vi "Cell Status Data File Functions.vi"(0 "FilePathIn":path=path "C:/ER2007/Cell Status.dat", 1 "Function":T3(ring), 2 "Cell Select - RO":i32, 3 "Keys":u16(ring) items=["Title", "Version", "Last Write", "CurCell", "NumCells", "Cell ID", "Status", "Project", "Sample ID", "Rock Type", "Fluid Pair", "Rw", "Rw Temp", "Length", "Diameter", "Porosity", "Permeability", "2P/4P", "Elect Spacing", "Frequency", "Amplitude", "DAQ Period", "DAQ Units", "Start Time", "Next Time", "Filename", "Pore Volume", "Pore Transducer", "Last Resistor", "ER 1-2", "ER 1-3", "ER 1-4", "ER 2-3", "FF 2-3", "Temp A", "Temp B", "Conf Press", "Pore Press", "Delta Press", "Pore Down"], 5 "Cell x Data In":T2 {"Rw Temp" format="%.2f"; "Rw" format="%.2f"; "DAQ Units" items=["Mins", "Hrs"]; "CurData" format="%.3f"; "Last Pore Vol" format="%.3f"; "Amplitude" format="%.3f"; "ElectSpace" format="%.2f"; "Permeability" format="%.2f"; "Porosity" format="%.2f"; "Diameter" format="%.2f"; "Length" format="%.2f"}, 7 "Cell ID List":i32[](array[numeric]), 11 "ErrorIn":errorcluster, 12 "Init w Values":bool, 13 "Version":string="1.00", 14 "Sections":u16(ring) items=["GenInfo", "Cell 1 Status", "Cell 2 Status", "Cell 3 Status", "Cell 4 Status", "Cell 5 Status"]) -> (4 "FilePathOut":path=path "C:/ER2007/Cell Status.dat", 6 "Cell x Data Out":T2 {"Rw Temp" format="%.2f"; "Rw" format="%.2f"; "DAQ Units" items=["Mins", "Hrs"]; "CurData" format="%.3f"; "Last Pore Vol" format="%.3f"; "Amplitude" format="%.3f"; "ElectSpace" format="%.2f"; "Permeability" format="%.2f"; "Porosity" format="%.2f"; "Diameter" format="%.2f"; "Length" format="%.2f"}, 8 "GenInfoOut":T1, 10 "Section Strings":string[](array[string])=["GenInfo", "Cell 1 Status", "Cell 2 Status", "Cell 3 Status", "Cell 4 Status", "Cell 5 Status"], 15 "ErrorOut":errorcluster)   [LabVIEW 2013]
uses:
  <vilib>/Utility/config.llb/Write Key (String).vi
  <vilib>/Utility/config.llb/Read Key (String).vi
  <vilib>/Utility/config.llb/NI_LVConfig.lvlib
panel:
  in  "Chop Keys at Index":i32=40
  out "Labels":string[](array[string])=["Cell ID", "Status", "Project", "Sample ID", "Rock Type", "Fluid Pair", "Rw", "Rw Temp", "Length", "Diameter", "Porosity", "Permeability", "2P/4P", "Elect Spacing", "Frequency", "Amplitude", "DAQ Period", "DAQ Units", "Start Time", "Next Time", "Filename", "Pore Volume", "Pore Transducer", "Last Resistor", " ER 1-2", "ER 1-3", "ER 1-4", "ER 2-3", "FF 2-3", "Temp A", "Temp B", "Conf Press", "Pore Press", "Delta Press", "Pore Down"]
  out "ErrorOut 2":errorcluster
  in  "SetStrings":bool
  # "Specific to ER2007 Cell Status Functions"
  # "To set the strings, the file must not exist.\nSet Function to \"New File\", \"Set Strings\"\nto ON, and run vi.  After running, make\ncurrent values default for \"Sections\",\n\"Keys\", and \"Section Strings\"."
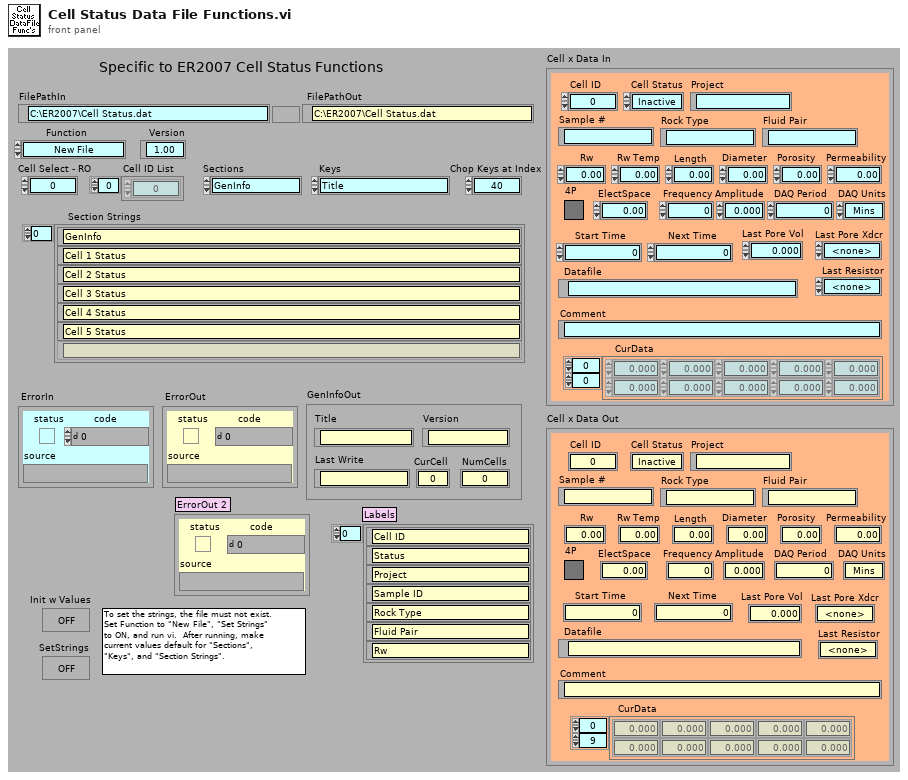
[diagram p1: front panel]
types:
  T1 = cluster{"Title":string, "Version":string, "Last Write":string, "CurCell":i32, "NumCells":i32}
  T2 = cluster{"Cell ID":i32, "Cell Status":enum16{"Inactive", "Setup", "Active", "Done"}, "Project":string, "Sample #":string, "Rock Type":string, "Fluid Pair":string, "Rw":dbl, "Rw Temp":dbl, "Length":dbl, "Diameter":dbl, "Porosity":dbl, "Permeability":dbl, "4P":bool, "ElectSpace":dbl, "Frequency":dbl, "Amplitude":dbl, "DAQ Period":u32, "DAQ Units":u16, "Start Time":dbl, "Next Time":dbl, "Datafile":path, "Last Pore Vol":dbl, "Last Pore Xdcr":enum16{"<none>", "Lo Range", "Hi Range"}, "Last Resistor":enum16{"<none>", "Resistor 1", "Resistor 2", "Resistor 3", "Resistor 4", "Resistor 5", "Resistor 6"}, "CurData":dbl[][], "Comment":string}
  T3 = enum16{"New File", "Read Cell Status", "Write Cell Status"}
  T4 = enum16{"<none>", "Resistor 1", "Resistor 2", "Resistor 3", "Resistor 4", "Resistor 5", "Resistor 6"}
  T5 = typedef "NI_LVConfig.lvlib/Config Data RefNum.ctl" = refnum<k1>
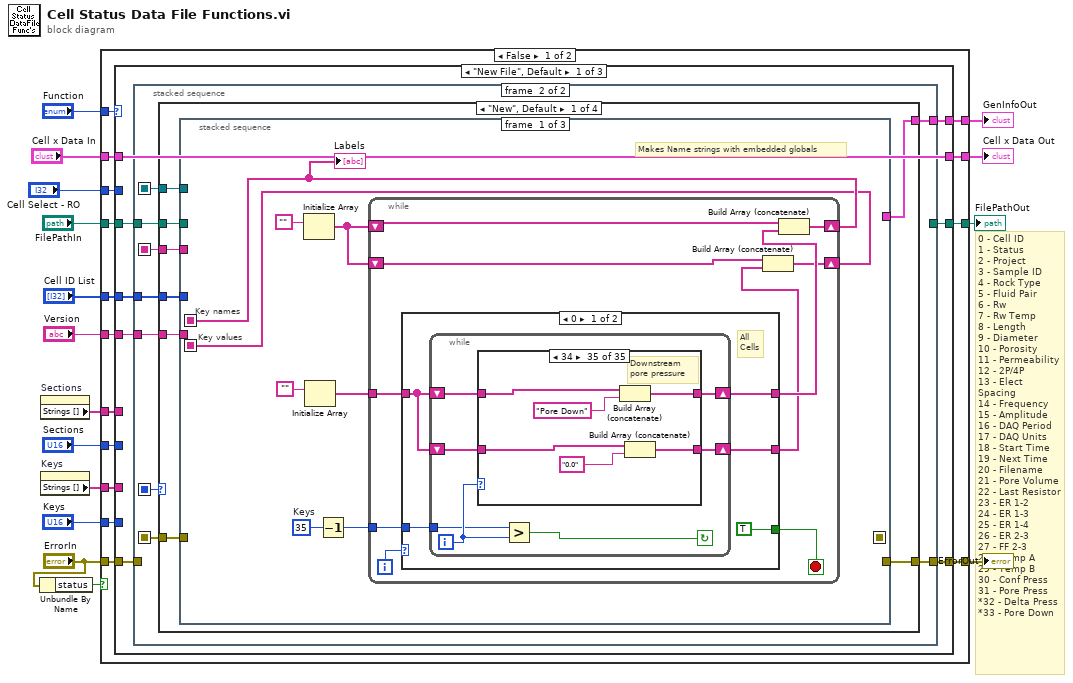
[diagram p0: block diagram]
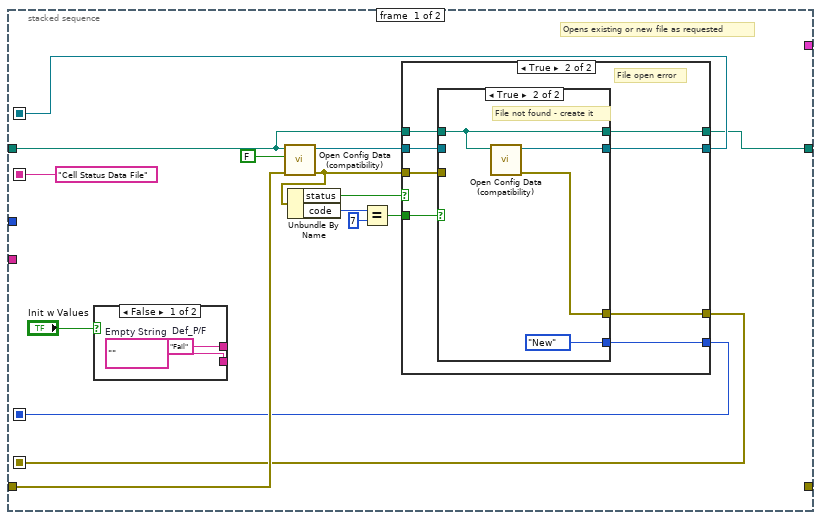
[diagram p2: hidden frame]
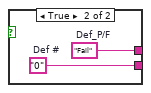
[diagram p3: hidden frame]
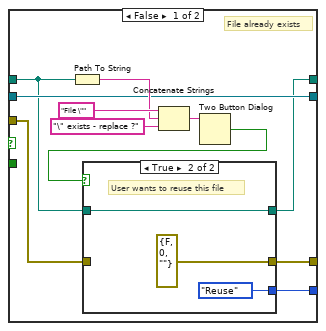
[diagram p4: hidden frame]
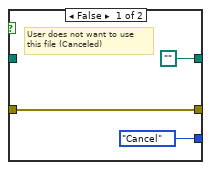
[diagram p5: hidden frame]
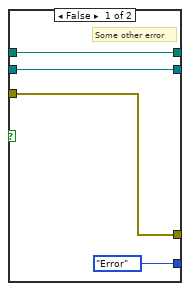
[diagram p6: hidden frame]
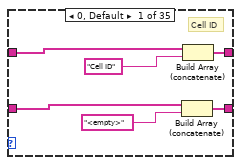
[diagram p7: hidden frame]
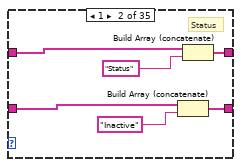
[diagram p8: hidden frame]
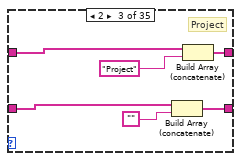
[diagram p9: hidden frame]
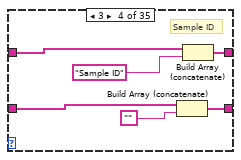
[diagram p10: hidden frame]
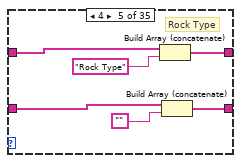
[diagram p11: hidden frame]
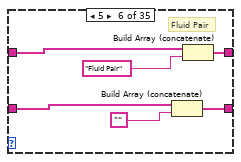
[diagram p12: hidden frame]
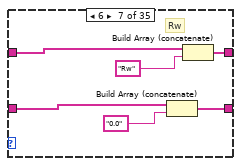
[diagram p13: hidden frame]
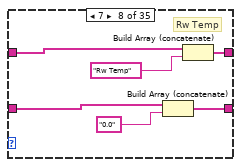
[diagram p14: hidden frame]
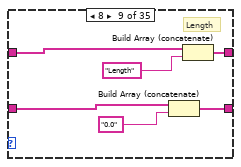
[diagram p15: hidden frame]
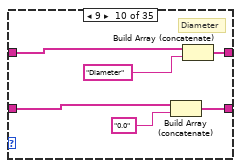
[diagram p16: hidden frame]
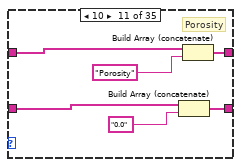
[diagram p17: hidden frame]
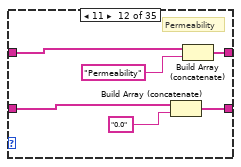
[diagram p18: hidden frame]
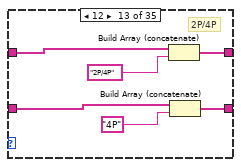
[diagram p19: hidden frame]
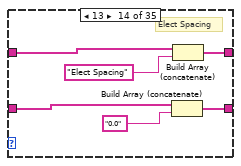
[diagram p20: hidden frame]
diagram:
  # "0 - Cell ID\n1 - Status\n2 - Project\n3 - Sample ID\n4 - Rock Type\n5 - Fluid Pair\n6 - Rw\n7 - Rw Temp\n8 - Length\n9 - Diameter\n10 - Porosity\n11 - Permeability\n12 - 2P/4P\n13 - Elect Spacing\n14 - Frequency\n15 - Amplitude\n16 - DAQ Period\n17 - DAQ Units\n18 - Start Time\n19 - Next Time\n20 - Filename\n21 - Pore Volume\n22 - Last Resistor\n23 - ER 1-2\n24 - ER 1-3\n25 - ER 1-4\n26 - ER 2-3\n27 - FF 2-3\n28 - Temp A\n29 - Temp B\n30 - Conf Press\n31 - Pore Press\n*32 - Delta Press\n*33 - Pore Down"
  n1 = Unbundle By Name("ErrorIn") -> ("status"=w16:bool)
  n2 = property on="Sections" class="Ring (strict)"() -> ("Strings []"=w11:string[])  [unwired: 2 in, 2 out]
  n3 = property on="Keys" class="Ring (strict)"() -> ("Strings []"=w9:string[])  [unwired: 2 in, 2 out]
  n4 = case shown="False" w16 {
    tunnel: "ErrorIn" -> [w29 w2061]
    tunnel: [w28 w2061] -> w14
    tunnel: "Function" -> [w31 _]
    tunnel: "FilePathIn" -> [w30 w2060]
    tunnel: "Cell ID List" -> [w27 _]
    tunnel: w11 -> [w26 _]
    tunnel: "Sections" -> [w25 _]
    tunnel: w9 -> [w24 _]
    tunnel: "Keys" -> [w23 _]
    tunnel: [w20 w2059] -> w4
    tunnel: [w22 w2060] -> w7
    tunnel: "Version" -> [w21 _]
    tunnel: "Cell x Data In" -> [w19 w2059]
    tunnel: "Cell Select - RO" -> [w18 _]
    tunnel: [w17 w2058] -> w1
    frame False {
      n5 = case shown="\"New File\", Default" w31 {
        tunnel: w30 -> [w39 w565 w1601]
        tunnel: w29 -> [w38 w577 w1612]
        tunnel: [w37 w573 w1609] -> w28
        tunnel: w27 -> [w36 _ _]
        tunnel: w26 -> [_ w567 w1604]
        tunnel: w25 -> [_ _ _]
        tunnel: w24 -> [_ w575 w1593]
        tunnel: w23 -> [_ _ _]
        tunnel: [w35 w565 w1601] -> w22
        tunnel: w21 -> [w34 _ w1592]
        tunnel: [w33 w557 w1591] -> w20
        tunnel: w19 -> [w33 w558 w1591]
        tunnel: w18 -> [_ w554 _]
        tunnel: [w32 w552 w1590] -> w17
        frame "New File", Default {
          n6 = stacked-sequence {
            seq-local: [w46 _] -> [_ w99]
            seq-local: [w44 _] -> [_ w98]
            seq-local: [w43 _] -> [_ w100]
            seq-local: ["Cell Status Data File" _] -> [_ w93]
            tunnel: w39 -> [w50 w95]
            tunnel: w38 -> [w53 _]
            tunnel: [_ w96] -> w37
            tunnel: w36 -> [_ w97]
            tunnel: [w42 _] -> w35
            tunnel: w34 -> [_ w94]
            tunnel: [_ w92] -> w32
            frame #0 {
              # "Opens existing or new file as requested"
              n7 = case shown="False" "Init w Values" {
                tunnel: [w56 w58] -> _
                tunnel: [w55 w57] -> _
                frame False {
                  w55 = ""  # Empty String
                  w56 = "Fail"  # Def_P/F
                }
                frame True {
                  w57 = "0"  # Def #
                  w58 = "Fail"  # Def_P/F
                }
              }
              n8 = call <vilib>:"Open Config Data (compatibility).vi"("error in (no error)"=w53, "create file if necessary (T)"=FALSE ("create file if necessary? (T)"), "configuration file path"=w50) -> ("error out"=w45:errorcluster, "refnum"=w51:T5)  [unwired: 6 in, 1 out]
              n9 = Unbundle By Name(w45) -> ("status"=w52:bool, "code"=w48:i32)
              n10 = Equal?(x=w48, y=7) -> (x = y?=w47:bool)
              n11 = case shown="True" w52 {
                tunnel: w51 -> [w62 w83]
                tunnel: w50 -> [w59 w78]
                tunnel: w47 -> [_ w79]
                tunnel: [w62 w82] -> w46
                tunnel: [w64 w80] -> w44
                tunnel: w45 -> [w63 w81]
                tunnel: [w61 w77] -> w43
                tunnel: [w60 w76] -> w42
                frame False {
                  # "File already exists"
                  n12 = Path To String(path=w59) -> (string=w68:string)
                  n13 = Concatenate Strings("File \"" ("message"), w68, "\" exists - replace ?" ("Substring")) -> (w66:string)
                  n14 = Two Button Dialog(message=w66) -> (T button?=w65:bool)  [unwired: 2 in]
                  n15 = case shown="True" w65 {
                    tunnel: [w72 errorcluster {"status"=FALSE, "code"=0, "source"=""} ("error out")] -> w64
                    tunnel: w63 -> [w72 _]
                    tunnel: [enum16{"New", "Reuse", "Error", "Cancel"}."Cancel" enum16{"New", "Reuse", "Error", "Cancel"}."Reuse"] -> w61
                    tunnel: w59 -> [_ w74]
                    tunnel: [path "" w74] -> w60
                    frame False {
                      # "User does not want to use\nthis file (Canceled)"
                    }
                    frame True {
                      # "User wants to reuse this file"
                    }
                  }
                }
                frame True {
                  # "File open error"
                  n16 = case shown="True" w79 {
                    tunnel: w83 -> [w87 _]
                    tunnel: [w87 w91] -> w82
                    tunnel: w81 -> [w86 _]
                    tunnel: [w86 w90] -> w80
                    tunnel: w78 -> [w85 w89]
                    tunnel: [enum16{"New", "Reuse", "Error", "Cancel"}."Error" enum16{"New", "Reuse", "Error", "Cancel"}."New"] -> w77
                    tunnel: [w85 w89] -> w76
                    frame False {
                      # "Some other error"
                    }
                    frame True {
                      # "File not found - create it"
                      n17 = call <vilib>:"Open Config Data (compatibility).vi"("configuration file path"=w89) -> ("error out"=w90:errorcluster, "refnum"=w91:T5)  [unwired: 8 in, 1 out]
                    }
                  }
                }
              }
            }
            frame #1 {
              n18 = case shown="\"New\", Default" w100 {
                tunnel: w99 -> [w108 w517 _ _]
                tunnel: w98 -> [w107 w516 w525 w530]
                tunnel: w97 -> [w106 _ _ _]
                tunnel: [w105 w513 w524 w529] -> w96
                tunnel: w95 -> [w104 _ _ _]
                tunnel: w94 -> [w103 w502 _ _]
                tunnel: w93 -> [w102 w503 _ _]
                tunnel: [w101 w500 w520 w531] -> w92
                frame "New", Default {
                  n19 = stacked-sequence {
                    seq-local: [w113 _ _] -> [_ w356 _]
                    seq-local: [_ w355 _] -> [_ _ w456]
                    seq-local: [w109 _ _] -> [_ w353 _]
                    tunnel: w108 -> [_ w360 w458]
                    tunnel: w107 -> [_ w357 _]
                    tunnel: w106 -> [_ w359 _]
                    tunnel: [_ _ w461] -> w105
                    tunnel: w104 -> [_ _ w457]
                    tunnel: w103 -> [_ w358 _]
                    tunnel: w102 -> [_ w354 _]
                    tunnel: [_ w352 _] -> w101
                    frame #0 {
                      w112 = 35  # Keys
                      # "Key values"
                      # "Key names"
                      # "Makes Name strings with embedded globals"
                      n20 = Initialize Array("") -> (w110:string[])  [unwired: 1 in]
                      n21 = Initialize Array("") -> (w114:string[])  [unwired: 1 in]
                      n22 = Decrement(x=w112) -> (x-1=w111:i32)
                      n23 = while {
                        shift-right: [w125] -> w113
                        shift-left: w110 -> [w126]
                        tunnel: w114 -> [w122]
                        tunnel: w111 -> [w120]
                        shift-right: [w118] -> w109
                        shift-left: w110 -> [w119]
                        i -> [w121]
                        stop <- w124 stop-if-true
                        n24 = case shown="0" w121 {
                          tunnel: [TRUE TRUE] -> w124
                          tunnel: [w130 w349] -> w123
                          tunnel: w122 -> [w128 _]
                          tunnel: w120 -> [w129 _]
                          tunnel: [w127 w349] -> w117
                          frame 0 {
                            # "All\nCells"
                            n25 = while {
                              shift-right: [w136] -> w130
                              shift-left: w128 -> [w135]
                              tunnel: w129 -> [w137]
                              shift-right: [w133] -> w127
                              shift-left: w128 -> [w132]
                              i -> [w138]
                              stop <- w134 continue-if-true
                              n26 = case shown="34" w138 {
                                tunnel: [w144 w150 w156 w162 w168 w174 w180 w186 w192 w198 w204 w210 w216 w222 w228 w234 w240 w246 w252 w258 w264 w270 w276 w282 w288 w294 w300 w306 w312 w318 w324 w330 w336 w342 w348] -> w136
                                tunnel: w135 -> [w143 w149 w155 w161 w167 w173 w179 w185 w191 w197 w203 w209 w215 w221 w227 w233 w239 w245 w251 w257 w263 w269 w275 w281 w287 w293 w299 w305 w311 w317 w323 w329 w335 w341 w347]
                                tunnel: [w140 w146 w153 w159 w165 w171 w176 w182 w188 w194 w200 w206 w212 w218 w224 w230 w236 w242 w248 w254 w260 w266 w272 w278 w284 w290 w296 w302 w308 w314 w320 w326 w332 w338 w344] -> w133
                                tunnel: w132 -> [w139 w145 w152 w158 w164 w170 w175 w181 w187 w193 w199 w205 w211 w217 w223 w229 w235 w241 w247 w253 w259 w265 w271 w277 w283 w289 w295 w301 w307 w313 w319 w325 w331 w337 w343]
                                frame 0, Default {
                                # "Cell ID"
                                n27 = Build Array (concatenate)(w139, "<empty>") -> (w140:string[])
                                n28 = Build Array (concatenate)(w143, "Cell ID") -> (w144:string[])
                                }
                                frame 1 {
                                # "Status"
                                n29 = Build Array (concatenate)(w145, "Inactive") -> (w146:string[])
                                n30 = Build Array (concatenate)(w149, "Status") -> (w150:string[])
                                }
                                frame 2 {
                                # "Project"
                                n31 = Build Array (concatenate)(w152, "") -> (w153:string[])
                                n32 = Build Array (concatenate)(w155, "Project") -> (w156:string[])
                                }
                                frame 3 {
                                # "Sample ID"
                                n33 = Build Array (concatenate)(w158, "") -> (w159:string[])
                                n34 = Build Array (concatenate)(w161, "Sample ID") -> (w162:string[])
                                }
                                frame 4 {
                                # "Rock Type"
                                n35 = Build Array (concatenate)(w167, "Rock Type") -> (w168:string[])
                                n36 = Build Array (concatenate)(w164, "") -> (w165:string[])
                                }
                                frame 5 {
                                # "Fluid Pair"
                                n37 = Build Array (concatenate)(w170, "") -> (w171:string[])
                                n38 = Build Array (concatenate)(w173, "Fluid Pair") -> (w174:string[])
                                }
                                frame 6 {
                                # "Rw"
                                n39 = Build Array (concatenate)(w175, "0.0") -> (w176:string[])
                                n40 = Build Array (concatenate)(w179, "Rw") -> (w180:string[])
                                }
                                frame 7 {
                                # "Rw Temp"
                                n41 = Build Array (concatenate)(w181, "0.0") -> (w182:string[])
                                n42 = Build Array (concatenate)(w185, "Rw Temp") -> (w186:string[])
                                }
                                frame 8 {
                                # "Length"
                                n43 = Build Array (concatenate)(w187, "0.0") -> (w188:string[])
                                n44 = Build Array (concatenate)(w191, "Length") -> (w192:string[])
                                }
                                frame 9 {
                                # "Diameter"
                                n45 = Build Array (concatenate)(w193, "0.0") -> (w194:string[])
                                n46 = Build Array (concatenate)(w197, "Diameter") -> (w198:string[])
                                }
                                frame 10 {
                                # "Porosity"
                                n47 = Build Array (concatenate)(w199, "0.0") -> (w200:string[])
                                n48 = Build Array (concatenate)(w203, "Porosity") -> (w204:string[])
                                }
                                frame 11 {
                                # "Permeability"
                                n49 = Build Array (concatenate)(w205, "0.0") -> (w206:string[])
                                n50 = Build Array (concatenate)(w209, "Permeability") -> (w210:string[])
                                }
                                frame 12 {
                                # "2P/4P"
                                n51 = Build Array (concatenate)(w215, "2P/4P") -> (w216:string[])
                                n52 = Build Array (concatenate)(w211, "4P") -> (w212:string[])
                                }
                                frame 13 {
                                # "Elect Spacing"
                                n53 = Build Array (concatenate)(w217, "0.0") -> (w218:string[])
                                n54 = Build Array (concatenate)(w221, "Elect Spacing") -> (w222:string[])
                                }
                                frame 14 {
                                # "Frequency"
                                n55 = Build Array (concatenate)(w227, "Frequency") -> (w228:string[])
                                n56 = Build Array (concatenate)(w223, "0.0") -> (w224:string[])
                                }
                                frame 15 {
                                # "Amplitude"
                                n57 = Build Array (concatenate)(w233, "Amplitude") -> (w234:string[])
                                n58 = Build Array (concatenate)(w229, "0.0") -> (w230:string[])
                                }
                                frame 16 {
                                # "DAQ Period"
                                n59 = Build Array (concatenate)(w239, "DAQ Period") -> (w240:string[])
                                n60 = Build Array (concatenate)(w235, "0.0") -> (w236:string[])
                                }
                                frame 17 {
                                # "DAQ Units"
                                n61 = Build Array (concatenate)(w241, "Hrs") -> (w242:string[])
                                n62 = Build Array (concatenate)(w245, "DAQ Units") -> (w246:string[])
                                }
                                frame 18 {
                                # "Start Time"
                                n63 = Build Array (concatenate)(w251, "Start Time") -> (w252:string[])
                                n64 = Build Array (concatenate)(w247, "0.0") -> (w248:string[])
                                }
                                frame 19 {
                                # "Next Time"
                                n65 = Build Array (concatenate)(w253, "0.0") -> (w254:string[])
                                n66 = Build Array (concatenate)(w257, "Next Time") -> (w258:string[])
                                }
                                frame 20 {
                                # "Filename"
                                n67 = Build Array (concatenate)(w259, "<Not A Path>") -> (w260:string[])
                                n68 = Build Array (concatenate)(w263, "Filename") -> (w264:string[])
                                }
                                frame 21 {
                                # "Pore Volume"
                                n69 = Build Array (concatenate)(w269, "Pore Volume") -> (w270:string[])
                                n70 = Build Array (concatenate)(w265, "0.0") -> (w266:string[])
                                }
                                frame 22 {
                                # "Pore Xdcr"
                                n71 = Build Array (concatenate)(w275, "Pore Transducer") -> (w276:string[])
                                n72 = Build Array (concatenate)(w271, "<none>") -> (w272:string[])
                                }
                                frame 23 {
                                # "Last Resistor"
                                n73 = Build Array (concatenate)(w281, "Last Resistor") -> (w282:string[])
                                n74 = Build Array (concatenate)(w277, "<none>") -> (w278:string[])
                                }
                                frame 24 {
                                # "ER 1-2"
                                n75 = Build Array (concatenate)(w283, "0.0") -> (w284:string[])
                                n76 = Build Array (concatenate)(w287, " ER 1-2") -> (w288:string[])
                                }
                                frame 25 {
                                # "ER 1-3"
                                n77 = Build Array (concatenate)(w293, "ER 1-3") -> (w294:string[])
                                n78 = Build Array (concatenate)(w289, "0.0") -> (w290:string[])
                                }
                                frame 26 {
                                # "ER 1-4"
                                n79 = Build Array (concatenate)(w299, "ER 1-4") -> (w300:string[])
                                n80 = Build Array (concatenate)(w295, "0.0") -> (w296:string[])
                                }
                                frame 27 {
                                # "ER 2-3"
                                n81 = Build Array (concatenate)(w305, "ER 2-3") -> (w306:string[])
                                n82 = Build Array (concatenate)(w301, "0.0") -> (w302:string[])
                                }
                                frame 28 {
                                # "FF 2-3"
                                n83 = Build Array (concatenate)(w307, "0.0") -> (w308:string[])
                                n84 = Build Array (concatenate)(w311, "FF 2-3") -> (w312:string[])
                                }
                                frame 29 {
                                # "Temp A"
                                n85 = Build Array (concatenate)(w317, "Temp A") -> (w318:string[])
                                n86 = Build Array (concatenate)(w313, "0.0") -> (w314:string[])
                                }
                                frame 30 {
                                # "Temp B"
                                n87 = Build Array (concatenate)(w323, "Temp B") -> (w324:string[])
                                n88 = Build Array (concatenate)(w319, "0.0") -> (w320:string[])
                                }
                                frame 31 {
                                # "Conf Press"
                                n89 = Build Array (concatenate)(w325, "0.0") -> (w326:string[])
                                n90 = Build Array (concatenate)(w329, "Conf Press") -> (w330:string[])
                                }
                                frame 32 {
                                # "Pore Press"
                                n91 = Build Array (concatenate)(w335, "Pore Press") -> (w336:string[])
                                n92 = Build Array (concatenate)(w331, "0.0") -> (w332:string[])
                                }
                                frame 33 {
                                # "Delta Press"
                                n93 = Build Array (concatenate)(w341, "Delta Press") -> (w342:string[])
                                n94 = Build Array (concatenate)(w337, "0.0") -> (w338:string[])
                                }
                                frame 34 {
                                # "Downstream\npore pressure"
                                n95 = Build Array (concatenate)(w347, "Pore Down") -> (w348:string[])
                                n96 = Build Array (concatenate)(w343, "0.0") -> (w344:string[])
                                }
                              }
                              n97 = Greater?(x=w137, y=w138) -> (0:w134:bool)
                            }
                          }
                          frame Default {
                            n98 = Build Array("<bad CASE in Cell Status Data File Functions.vi>") -> (w349:string[])
                          }
                        }
                        n99 = Build Array (concatenate)(w119, w117) -> (w118:string[])
                        n100 = Build Array (concatenate)(w126, w123) -> (w125:string[])
                      }
                      "Labels" <- w113
                    }
                    frame #1 {
                      n101 = while {
                        tunnel: w360 -> [w372]
                        tunnel: w359 -> [w371]
                        tunnel: w358 -> [w370]
                        shift-right: [w368] -> w355
                        shift-left: w357 -> [w369]
                        tunnel: w356 -> [w367]
                        tunnel: w354 -> [w366]
                        tunnel: w353 -> [w364]
                        shift-right: [w362] -> w352
                        shift-left: _ -> [w361]
                        i -> [w363]
                        stop <- w365 stop-if-true
                        n102 = case shown="1" w363 {
                          tunnel: w372 -> [w397 w400]
                          tunnel: w371 -> [_ w405]
                          tunnel: w370 -> [w382 _]
                          tunnel: w369 -> [w389 w403]
                          tunnel: [w377 w402] -> w368
                          tunnel: w367 -> [_ w404]
                          tunnel: w366 -> [w383 _]
                          tunnel: [FALSE w399] -> w365
                          tunnel: w364 -> [_ w401]
                          tunnel: [w380 w398] -> w362
                          tunnel: w361 -> [_ w398]
                          frame 0, Default {
                            w379 = T1 {"Title"="", "Version"="", "Last Write"="", "CurCell"=1, "NumCells"=5}  # GenInfoOut
                            w376 = "GenInfo" ("section")
                            # "GenInfo Section"
                            n103 = call-poly <vilib>:"Write Key.vi"("section"=w376, "error in (no error)"=w389, "value"=w383, "key"="Title", "refnum"=w397) -> ("error out"=w394:errorcluster, "refnum out"=w395:T5)  [unwired: 4 in, 1 out]
                            n104 = Get Date/Time String() -> (date string=w381:string)  [unwired: 3 in, 1 out]
                            n105 = call-poly <vilib>:"Write Key.vi"("section"=w376, "error in (no error)"=w394, "value"=w382, "key"="Version", "refnum"=w395) -> ("error out"=w392:errorcluster, "refnum out"=w391:T5)  [unwired: 4 in, 1 out]
                            n106 = call-poly <vilib>:"Write Key.vi"("section"=w376, "error in (no error)"=w392, "value"=w381, "key"="Last Write", "refnum"=w391) -> ("error out"=w387:errorcluster, "refnum out"=w386:T5)  [unwired: 4 in, 1 out]
                            n107 = Bundle By Name(cluster=w379, "Title"=w383, "Version"=w382, "Last Write"=w381) -> (w380:T1)
                            n108 = call-poly <vilib>:"Write Key.vi"("section"=w376, "error in (no error)"=w387, "value"="1" ("key"), "key"="CurCell", "refnum"=w386) -> ("error out"=w378:errorcluster, "refnum out"=w374:T5)  [unwired: 4 in, 1 out]
                            n109 = call-poly <vilib>:"Write Key.vi"("section"=w376, "error in (no error)"=w378, "value"="5" ("key"), "key"="NumCells", "refnum"=w374) -> ("error out"=w377:errorcluster)  [unwired: 4 in, 2 out]
                          }
                          frame 1 {
                            # "Makes the six cell info sections"
                            n110 = stacked-sequence {
                              seq-local: [w406 _] -> [_ w431]
                              seq-local: [w407 _] -> [_ w432]
                              tunnel: w405 -> [w409 _]
                              tunnel: w404 -> [_ w429]
                              tunnel: w403 -> [_ w434]
                              tunnel: [_ w433] -> w402
                              tunnel: w401 -> [_ w430]
                              tunnel: w400 -> [_ w428]
                              tunnel: [_ TRUE] -> w399
                              frame #0 {
                                # "Section Names"
                                # "Cell ID"
                                # "Gets the Cell ID list"
                                n111 = Array Size(array=w409) -> (size(s)=w411:i32)
                                n112 = Less Or Equal To 0?(x=w411) -> (x <= 0?=w410:bool)
                                n113 = case shown="True" w410 {
                                tunnel: w409 -> [w425 _]
                                tunnel: [w425 i32[] [1, 2, 3, 4, 5] ("Cell ID List")] -> w408
                                frame False {
                                }
                                frame True {
                                }
                                }
                                n114 = for {
                                tunnel: w408 -> [w414] mode=indexing
                                tunnel: [w413] -> w406 mode=indexing
                                tunnel: [w412] -> w407 mode=indexing
                                # "Cell ID"
                                # "Section Names"
                                n115 = case shown="1, Default" w414 {
                                tunnel: ["1" "2" "3" "4" "5"] -> w413
                                tunnel: ["Cell 1 Status" "Cell 2 Status" "Cell 3 Status" "Cell 4 Status" "Cell 5 Status"] -> w412
                                frame 1, Default {
                                }
                                frame 2 {
                                }
                                frame 3 {
                                }
                                frame 4 {
                                }
                                frame 5 {
                                }
                                }
                                }
                              }
                              frame #1 {
                                n116 = for {
                                tunnel: w432 -> [w441] mode=indexing
                                shift-right: [w439] -> w433
                                shift-left: w434 -> [w440]
                                tunnel: w431 -> [w438] mode=indexing
                                tunnel: w430 -> [w436]
                                tunnel: w429 -> [w437]
                                tunnel: w428 -> [w435]
                                # "Key values"
                                # "Key names"
                                # "Section Names"
                                # "Cell ID"
                                n117 = for {
                                tunnel: w437 -> [w444] mode=indexing
                                tunnel: w441 -> [w448]
                                shift-right: [w446] -> w439
                                shift-left: w440 -> [w447]
                                tunnel: w438 -> [w445]
                                tunnel: w436 -> [w443] mode=indexing
                                tunnel: w435 -> [w442]
                                i -> [w450]
                                n118 = case shown="1, Default" w450 {
                                tunnel: [w452 w455] -> w451
                                tunnel: [w453 w454] -> w449
                                tunnel: w445 -> [w453 _]
                                tunnel: w444 -> [w452 w455]
                                tunnel: w443 -> [_ w454]
                                frame 0 {
                                # "Cell ID is special"
                                }
                                frame 1, Default {
                                # "Most keys"
                                }
                                }
                                n119 = call-poly <vilib>:"Write Key.vi"("section"=w448, "error in (no error)"=w447, "value"=w449, "key"=w451, "refnum"=w442) -> ("error out"=w446:errorcluster)  [unwired: 4 in, 2 out]
                                }
                                }
                              }
                            }
                          }
                        }
                      }
                    }
                    frame #2 {
                      n120 = call <vilib>:"Close Config Data.vi"("error in (no error)"=w456, "write file if changed (T)"=TRUE ("write configuration file? (F)"), "refnum"=w458) -> ("error out"=w460:errorcluster)  [unwired: 7 in, 1 out]
                      n121 = case shown="True" "SetStrings" {
                        tunnel: w460 -> [w464 w477]
                        tunnel: [w464 w471] -> w459
                        tunnel: w457 -> [_ w476]
                        frame False {
                        }
                        frame True {
                          n122 = call <vilib>:"Open Config Data (compatibility).vi"("error in (no error)"=w477, "create file if necessary (T)"=FALSE ("create file if necessary? (T)"), "configuration file path"=w476) -> ("error out"=w474:errorcluster, "refnum"=w473:T5)  [unwired: 6 in, 1 out]
                          n123 = call <vilib>:"Get Section Names.vi"("error in (no error)"=w474, "refnum"=w473) -> ("error out"=w482:errorcluster, "section names"=w478:string[], "refnum out"=w479:T5)  [unwired: 7 in]
                          "Section Strings" <- w478
                          n124 = Initialize Array("") -> (w480:string[])  [unwired: 1 in]
                          n125 = property on="Sections" class="Ring (strict)"("Strings []"=w478) -> ()  [unwired: 2 in, 2 out]
                          n126 = Array Size(array=w478) -> (size(s)=w483:i32)
                          n127 = for {
                            N: w483 -> [_]
                            tunnel: w478 -> [w491] mode=indexing
                            shift-right: [w489] -> w470
                            shift-left: w482 -> [w490]
                            shift-right: [w486] -> w468
                            shift-left: w480 -> [w488]
                            tunnel: w479 -> [w485]
                            tunnel: [w484] -> w472
                            n128 = call <vilib>:"Get Key Names.vi"("section"=w491, "error in (no error)"=w490, "refnum"=w485) -> ("error out"=w489:errorcluster, "key names"=w487:string[], "refnum out"=w484:T5)  [unwired: 5 in, 1 out]
                            n129 = Build Array (concatenate)(w488, w487) -> (w486:string[])
                          }
                          n130 = call <vilib>:"Close Config Data.vi"("error in (no error)"=w470, "write file if changed (T)"=FALSE ("write configuration file? (T)"), "refnum"=w472) -> ("error out"=w471:errorcluster)  [unwired: 7 in, 1 out]
                          n131 = Array Subset(array=w468, index=0, length="Chop Keys at Index") -> (w466:string[])
                          n132 = property on="Keys" class="Ring (strict)"("Strings []"=w466) -> ()  [unwired: 2 in, 2 out]
                        }
                      }
                      n133 = call <vilib>:"Simple Error Handler.vi"("error in (no error)"=w459) -> ("error out"=w461:errorcluster)  [unwired: 4 in, 4 out]
                    }
                  }
                }
                frame "Reuse" {
                  w499 = T1 {"Title"="", "Version"="", "Last Write"="", "CurCell"=1, "NumCells"=5}  # GenInfoOut
                  w494 = "GenInfo" ("section")
                  # "Reuse file"
                  n134 = call-poly <vilib>:"Write Key.vi"("section"=w494, "error in (no error)"=w516, "value"=w503, "key"="Title", "refnum"=w517) -> ("error out"=w518:errorcluster, "refnum out"=w519:T5)  [unwired: 4 in, 1 out]
                  n135 = call-poly <vilib>:"Write Key.vi"("section"=w494, "error in (no error)"=w518, "value"=w502, "key"="Version", "refnum"=w519) -> ("error out"=w511:errorcluster, "refnum out"=w512:T5)  [unwired: 4 in, 1 out]
                  n136 = Get Date/Time String() -> (date string=w501:string)  [unwired: 3 in, 1 out]
                  n137 = call-poly <vilib>:"Write Key.vi"("section"=w494, "error in (no error)"=w511, "value"=w501, "key"="Last Write", "refnum"=w512) -> ("error out"=w507:errorcluster, "refnum out"=w506:T5)  [unwired: 4 in, 1 out]
                  n138 = call-poly <vilib>:"Write Key.vi"("section"=w494, "error in (no error)"=w507, "value"="1" ("key"), "key"="CurCell", "refnum"=w506) -> ("error out"=w498:errorcluster, "refnum out"=w497:T5)  [unwired: 4 in, 1 out]
                  n139 = call-poly <vilib>:"Write Key.vi"("section"=w494, "error in (no error)"=w498, "value"="5" ("key"), "key"="NumCells", "refnum"=w497) -> ("error out"=w495:errorcluster, "refnum out"=w496:T5)  [unwired: 4 in, 1 out]
                  n140 = Bundle By Name(cluster=w499, "Title"=w503, "Version"=w502, "Last Write"=w501) -> (w500:T1)
                  n141 = call <vilib>:"Close Config Data.vi"("error in (no error)"=w495, "write file if changed (T)"=TRUE ("write configuration file? (F)"), "refnum"=w496) -> ("error out"=w514:errorcluster)  [unwired: 7 in, 1 out]
                  n142 = call <vilib>:"Simple Error Handler.vi"("error in (no error)"=w514) -> ("error out"=w513:errorcluster)  [unwired: 4 in, 4 out]
                }
                frame "Error" {
                  w520 = T1 {"Title"="", "Version"="", "Last Write"="", "CurCell"=1, "NumCells"=5}  # GenInfoOut
                  # "Error"
                  n143 = property class="VI"() -> ("VI Name"=w523:string)  [unwired: 2 in, 2 out]
                  n144 = Bundle By Name(cluster=w525, "status"=TRUE, "code"=6, "source"=w523) -> (w524:errorcluster)
                  "ErrorOut 2" <- w525
                }
                frame "Cancel" {
                  # "Canceled"
                  n145 = property class="VI"() -> ("VI Name"=w526:string)  [unwired: 2 in, 2 out]
                  n146 = local read "GenInfoOut"() -> (w531:T1)
                  n147 = Bundle By Name(cluster=w530, "status"=TRUE, "code"=43, "source"=w526) -> (w529:errorcluster)
                }
              }
            }
          }
        }
        frame "Read Cell Status" {
          w533 = T1 {"Title"="", "Version"="", "Last Write"="", "CurCell"=1, "NumCells"=5}  # GenInfoOut
          w534 = 4  # Add for CurData
          # "36"
          n148 = Unbundle By Name(w558) -> ("CurData"=w543:dbl[][])
          n149 = Array Subset(array=w575, index=0) -> (w553:string[])  [unwired: 1 in]
          n150 = call <vilib>:"Open Config Data (compatibility).vi"("error in (no error)"=w577, "create file if necessary (T)"=FALSE ("create file if necessary? (T)"), "configuration file path"=w565) -> ("error out"=w569:errorcluster, "refnum"=w568:T5)  [unwired: 6 in, 1 out]
          n151 = Array Size(array=w553) -> (size(s)=w566:i32)
          n152 = Array Size(array=w567) -> (size(s)=w555:i32)
          n153 = Initialize Array(0.0 ("element"), 15 ("dimension size")) -> (w540:dbl[])
          n154 = Decrement(x=w566) -> (x-1=w563:i32)
          n155 = case shown="1, Default" w554 {
            selector: w554 -> [_ w615]
            tunnel: [w583 w617] -> w550
            tunnel: w558 -> [w582 _]
            tunnel: w555 -> [w581 w616]
            frame 0 {
              n156 = Unbundle By Name(w582) -> ("Cell ID"=w585:i32)
              n157 = case shown="0, Default" w585 {
                selector: w585 -> [w589 w591 w595 w599 w603 _ _ _]
                tunnel: [w586 w590 w594 w598 w602 w608 w611 w613] -> w583
                tunnel: 1 -> [w587 w592 w596 w600 w604 w607 w610 w614]
                tunnel: w581 -> [_ _ _ _ _ w606 w609 w612]
                frame 0, Default {
                  n158 = To Long Integer(number=w589) -> (32bit integer=w588:i32)
                  n159 = Add(x=w588, y=w587) -> (x+y=w586:i32)
                }
                frame 1 {
                  n160 = To Long Integer(number=w591) -> (32bit integer=w593:i32)
                  n161 = Add(x=w593, y=w592) -> (x+y=w590:i32)
                }
                frame 2 {
                  n162 = To Long Integer(number=w595) -> (32bit integer=w597:i32)
                  n163 = Add(x=w597, y=w596) -> (x+y=w594:i32)
                }
                frame 3 {
                  n164 = To Long Integer(number=w599) -> (32bit integer=w601:i32)
                  n165 = Add(x=w601, y=w600) -> (x+y=w598:i32)
                }
                frame 4 {
                  n166 = To Long Integer(number=w603) -> (32bit integer=w605:i32)
                  n167 = Add(x=w605, y=w604) -> (x+y=w602:i32)
                }
                frame 5 {
                  n168 = Add(x=w606, y=w607) -> (x+y=w608:i32)
                }
                frame 6 {
                  n169 = Add(x=w609, y=w610) -> (x+y=w611:i32)
                }
                frame 7 {
                  n170 = Add(x=w612, y=w614) -> (x+y=w613:i32)
                }
              }
            }
            frame 1, Default {
              n171 = case shown="2" w615 {
                selector: w615 -> [w622 w624 w628 w632 w636]
                tunnel: [w619 w623 w627 w631 w635] -> w617
                tunnel: 0 -> [w620 w625 w629 w633 w637]
                tunnel: w616 -> [_ _ _ _ _]
                frame 1, Default {
                  n172 = To Long Integer(number=w622) -> (32bit integer=w621:i32)
                  n173 = Add(x=w621, y=w620) -> (x+y=w619:i32)
                }
                frame 2 {
                  n174 = To Long Integer(number=w624) -> (32bit integer=w626:i32)
                  n175 = Add(x=w626, y=w625) -> (x+y=w623:i32)
                }
                frame 3 {
                  n176 = To Long Integer(number=w628) -> (32bit integer=w630:i32)
                  n177 = Add(x=w630, y=w629) -> (x+y=w627:i32)
                }
                frame 4 {
                  n178 = To Long Integer(number=w632) -> (32bit integer=w634:i32)
                  n179 = Add(x=w634, y=w633) -> (x+y=w631:i32)
                }
                frame 5 {
                  n180 = To Long Integer(number=w636) -> (32bit integer=w638:i32)
                  n181 = Add(x=w638, y=w637) -> (x+y=w635:i32)
                }
              }
            }
          }
          n182 = Index Array(array=w567, index #1=0 ("index"), index #2=w550) -> (element #1=w548:string, element #2=w549:string)
          n183 = Index Array(array=w543, index (col)=0 ("disabled index (col)")) -> (element=w560:dbl[])  [unwired: 1 in]
          n184 = Add(x=w563, y=w534) -> (x+y=w535:i32)
          n185 = Array Size(array=w560) -> (size(s)=w559:i32)
          n186 = Decrement(x=w559) -> (x-1=w545:i32)
          n187 = Greater Than 0?(x=w545) -> (x > 0?=w536:bool)
          n188 = Index Array(array=w543, index (row)=w545) -> (element=w539:dbl[])  [unwired: 1 in]
          n189 = Select(t=w539, s=w536, f=w540) -> (s? t:f=w538:dbl[])
          n190 = while {
            shift-right: [w658] -> w572
            shift-left: w568 -> [w657]
            shift-right: [w661] -> w571
            shift-left: w569 -> [w660]
            tunnel: w549 -> [w656]
            tunnel: w553 -> [w649] mode=indexing
            tunnel: w535 -> [w654]
            shift-right: [w651] -> w556
            shift-left: w558 -> [w640]
            tunnel: [w650] -> w564
            tunnel: [w649] -> w551
            tunnel: [w648] -> w562
            shift-right: [w646] -> w537
            shift-left: w538 -> [w647]
            tunnel: w538 -> [w645]
            shift-right: [w643] -> w552
            shift-left: w533 -> [w644]
            tunnel: w548 -> [w642]
            tunnel: [w641] -> w546
            tunnel: w536 -> [w639]
            i -> [w655]
            stop <- w653 continue-if-true
            n191 = Greater?(x=w654, y=w655) -> (0:w652:bool)
            n192 = case shown="43" w655 {
              tunnel: [w677 w693 w709 w726 w743 w760 w781 w805 w821 w837 w853 w871 w889 w907 w925 w943 w961 w979 w997 w1015 w1033 w1051 w1067 w1095 w1113 w1130 w1148 w1165 w1185 w1210 w1239 w1268 w1297 w1326 w1355 w1384 w1413 w1442 w1471 w1500 w1519 w1535 w1551 w1566] -> w661
              tunnel: w660 -> [w676 w692 w708 w725 w742 w759 w780 w804 w820 w836 w852 w870 w888 w906 w924 w942 w960 w978 w996 w1014 w1032 w1050 w1066 w1094 w1112 w1129 w1147 w1164 w1184 w1209 w1238 w1267 w1296 w1325 w1354 w1383 w1412 w1441 w1470 w1499 w1519 w1535 w1551 w1566]
              tunnel: "" -> [w675 w691 w707 w724 w741 w758 w779 w803 w819 w835 w851 w869 w887 w905 w923 w941 w959 w977 w995 w1013 w1031 w1049 w1065 w1093 w1111 w1128 w1146 w1163 w1183 w1208 w1237 w1266 w1295 w1324 w1353 w1382 w1411 w1440 w1469 w1498 _ _ _ _]
              tunnel: [w674 w690 w706 w723 w740 w757 w778 w802 w818 w834 w850 w868 w886 w904 w922 w940 w958 w976 w994 w1012 w1030 w1048 w1064 w1092 w1110 w1127 w1145 w1162 w1182 w1207 w1236 w1265 w1294 w1323 w1352 w1381 w1410 w1439 w1468 w1497 w1517 w1533 w1549 w1564] -> w658
              tunnel: w657 -> [w673 w689 w705 w722 w739 w756 w777 w801 w817 w833 w849 w867 w885 w903 w921 w939 w957 w975 w993 w1011 w1029 w1047 w1063 w1091 w1109 w1126 w1144 w1161 w1181 w1206 w1235 w1264 w1293 w1322 w1351 w1380 w1409 w1438 w1467 w1496 w1517 w1533 w1549 w1564]
              tunnel: w656 -> [_ _ _ _ _ w747 w767 w791 w807 w823 w839 w855 w873 w891 w909 w927 w945 w963 w981 w999 w1017 w1035 w1053 w1080 w1097 w1115 w1132 w1150 w1170 w1194 w1223 w1252 w1281 w1310 w1339 w1368 w1397 w1427 w1456 w1485 _ _ _ _]
              tunnel: [w670 w686 w702 w719 w736 w752 w772 w797 w812 w828 w844 w864 w882 w900 w918 w936 w954 w971 w990 w1008 w1026 w1043 w1059 w1088 w1106 w1122 w1141 w1158 w1178 w1204 w1233 w1262 w1291 w1320 w1349 w1378 w1407 w1425 w1454 w1483 TRUE ("found?") TRUE ("found?") TRUE ("found?") TRUE ("found?")] -> w650
              tunnel: w649 -> [w672 w688 w704 w721 w738 w755 w776 w800 w816 w832 w848 w866 w884 w902 w920 w938 w956 w974 w992 w1010 w1028 w1046 w1062 w1090 w1108 w1125 w1143 w1160 w1180 w1205 w1234 w1263 w1292 w1321 w1350 w1379 w1408 w1437 w1466 w1495 _ _ _ _]
              tunnel: [w662 w678 w694 w712 w729 w754 w775 w799 w815 w831 w847 w865 w883 w901 w919 w937 w955 w973 w991 w1009 w1027 w1045 w1061 w1089 w1107 w1124 w1142 w1159 w1179 w1193 w1222 w1251 w1280 w1309 w1338 w1367 w1396 w1426 w1455 w1484 w1520 w1527 w1543 w1558] -> w651
              tunnel: [TRUE TRUE TRUE TRUE TRUE TRUE TRUE TRUE TRUE TRUE TRUE w860 w876 w895 w913 w931 w949 TRUE w985 w1003 w1021 TRUE TRUE w1084 w1101 TRUE w1136 TRUE TRUE w1202 w1231 w1260 w1289 w1318 w1347 w1376 w1405 w1435 w1464 w1493 TRUE TRUE TRUE TRUE] -> w648
              tunnel: w647 -> [w666 w682 w698 w716 w733 w749 w769 w793 w809 w825 w841 w857 w875 w893 w911 w929 w947 w965 w983 w1001 w1019 w1037 w1055 w1082 w1099 w1117 w1134 w1155 w1175 w1195 w1228 w1253 w1282 w1311 w1344 w1373 w1402 w1432 w1461 w1490 w1513 w1529 w1545 w1560]
              tunnel: [w666 w682 w698 w716 w733 w749 w769 w793 w809 w825 w841 w857 w875 w893 w911 w929 w947 w965 w983 w1001 w1019 w1037 w1055 w1082 w1099 w1117 w1134 w1155 w1175 w1201 w1230 w1259 w1288 w1317 w1346 w1375 w1404 w1434 w1463 w1492 w1512 w1528 w1544 w1559] -> w646
              tunnel: w645 -> [_ _ _ _ _ _ _ _ _ _ _ _ _ _ _ _ _ _ _ _ _ _ _ _ _ _ _ _ _ w1196 w1224 w1254 w1283 w1312 w1341 w1369 w1398 w1428 w1457 w1486 _ _ _ _]
              tunnel: w644 -> [w665 w681 w697 w715 w732 w748 w768 w792 w808 w824 w840 w856 w874 w892 w910 w928 w946 w964 w982 w1000 w1018 w1036 w1054 w1081 w1098 w1116 w1133 w1154 w1174 w1197 w1225 w1255 w1284 w1313 w1340 w1370 w1399 w1429 w1458 w1487 w1521 w1536 w1552 w1567]
              tunnel: [w664 w680 w696 w714 w731 w748 w768 w792 w808 w824 w840 w856 w874 w892 w910 w928 w946 w964 w982 w1000 w1018 w1036 w1054 w1081 w1098 w1116 w1133 w1154 w1174 w1197 w1225 w1255 w1284 w1313 w1340 w1370 w1399 w1429 w1458 w1487 w1521 w1536 w1552 w1567] -> w643
              tunnel: w642 -> [w663 w679 w695 w713 w730 _ _ _ _ _ _ _ _ _ _ _ _ _ _ _ _ _ _ _ _ _ _ _ _ _ _ _ _ _ _ _ _ _ _ _ _ _ _ _]
              tunnel: [w663 w679 w695 w713 w730 w747 w767 w791 w807 w823 w839 w855 w873 w891 w909 w927 w945 w963 w981 w999 w1017 w1035 w1053 w1080 w1097 w1115 w1132 w1150 w1170 w1194 w1223 w1252 w1281 w1310 w1339 w1368 w1397 w1427 w1456 w1485 "" "" "" ""] -> w641
              tunnel: w640 -> [w662 w678 w694 w712 w729 w746 w766 w790 w806 w822 w838 w854 w872 w890 w908 w926 w944 w962 w980 w998 w1016 w1034 w1052 w1079 w1096 w1114 w1131 w1149 w1169 w1193 w1222 w1251 w1280 w1309 w1338 w1367 w1396 w1426 w1455 w1484 w1520 w1527 w1543 w1558]
              tunnel: w639 -> [_ _ _ _ _ _ _ _ _ _ _ _ _ _ _ _ _ _ _ _ _ _ _ _ _ _ _ _ _ _ _ _ _ _ _ _ _ _ _ _ w1514 w1530 w1546 w1561]
              frame 0, Default {
                # "GenInfo - Title"
                n193 = call-poly <vilib>:"Read Key.vi"("section"=w663, "error in (no error)"=w676, "default value"=w675, "key"=w672, "refnum"=w673) -> ("error out"=w677:errorcluster, "value"=w669:string, "found?"=w670:bool, "refnum out"=w674:T5)  [unwired: 3 in]
                n194 = Unbundle By Name(w665) -> ("Title"=w668:string)
                n195 = Select(t=w669, s=w670, f=w668) -> (s? t:f=w671:string)
                n196 = Bundle By Name(cluster=w665, "Title"=w671) -> (w664:T1)
              }
              frame 1 {
                # "GenInfo - Version"
                n197 = call-poly <vilib>:"Read Key.vi"("section"=w679, "error in (no error)"=w692, "default value"=w691, "key"=w688, "refnum"=w689) -> ("error out"=w693:errorcluster, "value"=w685:string, "found?"=w686:bool, "refnum out"=w690:T5)  [unwired: 3 in]
                n198 = Unbundle By Name(w681) -> ("Version"=w684:string)
                n199 = Select(t=w685, s=w686, f=w684) -> (s? t:f=w687:string)
                n200 = Bundle By Name(cluster=w681, "Version"=w687) -> (w680:T1)
              }
              frame 2 {
                # "GenInfo - Last Write"
                n201 = call-poly <vilib>:"Read Key.vi"("section"=w695, "error in (no error)"=w708, "default value"=w707, "key"=w704, "refnum"=w705) -> ("error out"=w709:errorcluster, "value"=w701:string, "found?"=w702:bool, "refnum out"=w706:T5)  [unwired: 3 in]
                n202 = Unbundle By Name(w697) -> ("Last Write"=w700:string)
                n203 = Select(t=w701, s=w702, f=w700) -> (s? t:f=w703:string)
                n204 = Bundle By Name(cluster=w697, "Last Write"=w703) -> (w696:T1)
              }
              frame 3 {
                # "GenInfo - Current Cell"
                n205 = call-poly <vilib>:"Read Key.vi"("section"=w713, "error in (no error)"=w725, "default value"=w724, "key"=w721, "refnum"=w722) -> ("error out"=w726:errorcluster, "value"=w711:string, "found?"=w719:bool, "refnum out"=w723:T5)  [unwired: 3 in]
                n206 = Decimal String To Number(string=w711) -> (number=w710:i32)  [unwired: 2 in, 1 out]
                n207 = Unbundle By Name(w715) -> ("CurCell"=w718:i32)
                n208 = Select(t=w710, s=w719, f=w718) -> (s? t:f=w720:i32)
                n209 = Bundle By Name(cluster=w715, "CurCell"=w720) -> (w714:T1)
              }
              frame 4 {
                # "GenInfo - Num Cells"
                n210 = call-poly <vilib>:"Read Key.vi"("section"=w730, "error in (no error)"=w742, "default value"=w741, "key"=w738, "refnum"=w739) -> ("error out"=w743:errorcluster, "value"=w728:string, "found?"=w736:bool, "refnum out"=w740:T5)  [unwired: 3 in]
                n211 = Decimal String To Number(string=w728) -> (number=w727:i32)  [unwired: 2 in, 1 out]
                n212 = Unbundle By Name(w732) -> ("NumCells"=w735:i32)
                n213 = Select(t=w727, s=w736, f=w735) -> (s? t:f=w737:i32)
                n214 = Bundle By Name(cluster=w732, "NumCells"=w737) -> (w731:T1)
              }
              frame 5 {
                # "Cell Number"
                n215 = call-poly <vilib>:"Read Key.vi"("section"=w747, "error in (no error)"=w759, "default value"=w758, "key"=w755, "refnum"=w756) -> ("error out"=w760:errorcluster, "value"=w745:string, "found?"=w752:bool, "refnum out"=w757:T5)  [unwired: 3 in]
                n216 = Unbundle By Name(w746) -> ("Cell ID"=w751:i32)
                n217 = Decimal String To Number(string=w745) -> (number=w744:i32)  [unwired: 2 in, 1 out]
                n218 = case shown="True" w752 {
                  tunnel: w744 -> [_ w763]
                  tunnel: [w761 w762] -> w753
                  tunnel: w751 -> [w761 _]
                  frame False {
                    # "Key not found"
                  }
                  frame True {
                    n219 = case shown="1..5" w763 {
                      selector: w763 -> [_ w765]
                      tunnel: [1 w765] -> w762
                      frame Default {
                      }
                      frame 1..5 {
                      }
                    }
                  }
                }
                n220 = Bundle By Name(cluster=w746, "Cell ID"=w753) -> (w754:T2)
              }
              frame 6 {
                # "Cell Status"
                n221 = call-poly <vilib>:"Read Key.vi"("section"=w767, "error in (no error)"=w780, "default value"=w779, "key"=w776, "refnum"=w777) -> ("error out"=w781:errorcluster, "value"=w774:string, "found?"=w772:bool, "refnum out"=w778:T5)  [unwired: 3 in]
                n222 = Unbundle By Name(w766) -> ("Cell Status"=w771:enum16{"Inactive", "Setup", "Active", "Done"})
                n223 = case shown="True" w772 {
                  tunnel: w774 -> [_ w784]
                  tunnel: [w782 w783] -> w773
                  tunnel: w771 -> [w782 _]
                  frame False {
                    # "Key not found"
                  }
                  frame True {
                    n224 = case shown="\"Active\"" w784 {
                      tunnel: [enum16{"Inactive", "Setup", "Active", "Done"}."Inactive" ("Cell Status") enum16{"Inactive", "Setup", "Active", "Done"}."Inactive" ("Cell Status") enum16{"Inactive", "Setup", "Active", "Done"}."Setup" ("Cell Status") enum16{"Inactive", "Setup", "Active", "Done"}."Active" ("Cell Status") enum16{"Inactive", "Setup", "Active", "Done"}."Done" ("Cell Status")] -> w783
                      frame Default {
                      }
                      frame "Inactive" {
                      }
                      frame "Setup" {
                      }
                      frame "Active" {
                      }
                      frame "Done" {
                      }
                    }
                  }
                }
                n225 = Bundle By Name(cluster=w766, "Cell Status"=w773) -> (w775:T2)
              }
              frame 7 {
                # "Project"
                n226 = call-poly <vilib>:"Read Key.vi"("section"=w791, "error in (no error)"=w804, "default value"=w803, "key"=w800, "refnum"=w801) -> ("error out"=w805:errorcluster, "value"=w796:string, "found?"=w797:bool, "refnum out"=w802:T5)  [unwired: 3 in]
                n227 = Unbundle By Name(w790) -> ("Project"=w795:string)
                n228 = Select(t=w796, s=w797, f=w795) -> (s? t:f=w798:string)
                n229 = Bundle By Name(cluster=w790, "Project"=w798) -> (w799:T2)
              }
              frame 8 {
                # "Sample #"
                n230 = call-poly <vilib>:"Read Key.vi"("section"=w807, "error in (no error)"=w820, "default value"=w819, "key"=w816, "refnum"=w817) -> ("error out"=w821:errorcluster, "value"=w814:string, "found?"=w812:bool, "refnum out"=w818:T5)  [unwired: 3 in]
                n231 = Unbundle By Name(w806) -> ("Sample #"=w811:string)
                n232 = Select(t=w814, s=w812, f=w811) -> (s? t:f=w813:string)
                n233 = Bundle By Name(cluster=w806, "Sample #"=w813) -> (w815:T2)
              }
              frame 9 {
                # "Rock Type"
                n234 = call-poly <vilib>:"Read Key.vi"("section"=w823, "error in (no error)"=w836, "default value"=w835, "key"=w832, "refnum"=w833) -> ("error out"=w837:errorcluster, "value"=w830:string, "found?"=w828:bool, "refnum out"=w834:T5)  [unwired: 3 in]
                n235 = Unbundle By Name(w822) -> ("Rock Type"=w827:string)
                n236 = Select(t=w830, s=w828, f=w827) -> (s? t:f=w829:string)
                n237 = Bundle By Name(cluster=w822, "Rock Type"=w829) -> (w831:T2)
              }
              frame 10 {
                # "Fluid Pair"
                n238 = call-poly <vilib>:"Read Key.vi"("section"=w839, "error in (no error)"=w852, "default value"=w851, "key"=w848, "refnum"=w849) -> ("error out"=w853:errorcluster, "value"=w846:string, "found?"=w844:bool, "refnum out"=w850:T5)  [unwired: 3 in]
                n239 = Unbundle By Name(w838) -> ("Fluid Pair"=w843:string)
                n240 = Select(t=w846, s=w844, f=w843) -> (s? t:f=w845:string)
                n241 = Bundle By Name(cluster=w838, "Fluid Pair"=w845) -> (w847:T2)
              }
              frame 11 {
                # "Rw"
                n242 = call-poly <vilib>:"Read Key.vi"("section"=w855, "error in (no error)"=w870, "default value"=w869, "key"=w866, "refnum"=w867) -> ("error out"=w871:errorcluster, "value"=w862:string, "found?"=w864:bool, "refnum out"=w868:T5)  [unwired: 3 in]
                n243 = Unbundle By Name(w854) -> ("Rw"=w863:dbl)
                n244 = Fract/Exp String To Number(string=w862) -> (number=w861:dbl)  [unwired: 3 in, 1 out]
                n245 = Select(t=w861, s=w864, f=w863) -> (s? t:f=w859:dbl)
                n246 = Bundle By Name(cluster=w854, "Rw"=w859) -> (w865:T2)
                n247 = Not Equal?(x=w859, y=nan) -> (x != y?=w860:bool)
              }
              frame 12 {
                # "RW Temp"
                n248 = call-poly <vilib>:"Read Key.vi"("section"=w873, "error in (no error)"=w888, "default value"=w887, "key"=w884, "refnum"=w885) -> ("error out"=w889:errorcluster, "value"=w880:string, "found?"=w882:bool, "refnum out"=w886:T5)  [unwired: 3 in]
                n249 = Unbundle By Name(w872) -> ("Rw Temp"=w881:dbl)
                n250 = Fract/Exp String To Number(string=w880) -> (number=w879:dbl)  [unwired: 3 in, 1 out]
                n251 = Select(t=w879, s=w882, f=w881) -> (s? t:f=w877:dbl)
                n252 = Bundle By Name(cluster=w872, "Rw Temp"=w877) -> (w883:T2)
                n253 = Not Equal?(x=w877, y=nan) -> (x != y?=w876:bool)
              }
              frame 13 {
                # "Length"
                n254 = call-poly <vilib>:"Read Key.vi"("section"=w891, "error in (no error)"=w906, "default value"=w905, "key"=w902, "refnum"=w903) -> ("error out"=w907:errorcluster, "value"=w898:string, "found?"=w900:bool, "refnum out"=w904:T5)  [unwired: 3 in]
                n255 = Unbundle By Name(w890) -> ("Length"=w899:dbl)
                n256 = Fract/Exp String To Number(string=w898) -> (number=w897:dbl)  [unwired: 3 in, 1 out]
                n257 = Select(t=w897, s=w900, f=w899) -> (s? t:f=w894:dbl)
                n258 = Bundle By Name(cluster=w890, "Length"=w894) -> (w901:T2)
                n259 = Not Equal?(x=w894, y=nan) -> (x != y?=w895:bool)
              }
              frame 14 {
                # "Diameter"
                n260 = call-poly <vilib>:"Read Key.vi"("section"=w909, "error in (no error)"=w924, "default value"=w923, "key"=w920, "refnum"=w921) -> ("error out"=w925:errorcluster, "value"=w916:string, "found?"=w918:bool, "refnum out"=w922:T5)  [unwired: 3 in]
                n261 = Unbundle By Name(w908) -> ("Diameter"=w917:dbl)
                n262 = Fract/Exp String To Number(string=w916) -> (number=w915:dbl)  [unwired: 3 in, 1 out]
                n263 = Select(t=w915, s=w918, f=w917) -> (s? t:f=w912:dbl)
                n264 = Bundle By Name(cluster=w908, "Diameter"=w912) -> (w919:T2)
                n265 = Not Equal?(x=w912, y=nan) -> (x != y?=w913:bool)
              }
              frame 15 {
                # "Porosity"
                n266 = call-poly <vilib>:"Read Key.vi"("section"=w927, "error in (no error)"=w942, "default value"=w941, "key"=w938, "refnum"=w939) -> ("error out"=w943:errorcluster, "value"=w934:string, "found?"=w936:bool, "refnum out"=w940:T5)  [unwired: 3 in]
                n267 = Unbundle By Name(w926) -> ("Porosity"=w935:dbl)
                n268 = Fract/Exp String To Number(string=w934) -> (number=w933:dbl)  [unwired: 3 in, 1 out]
                n269 = Select(t=w933, s=w936, f=w935) -> (s? t:f=w930:dbl)
                n270 = Bundle By Name(cluster=w926, "Porosity"=w930) -> (w937:T2)
                n271 = Not Equal?(x=w930, y=nan) -> (x != y?=w931:bool)
              }
              frame 16 {
                # "Permeability"
                n272 = call-poly <vilib>:"Read Key.vi"("section"=w945, "error in (no error)"=w960, "default value"=w959, "key"=w956, "refnum"=w957) -> ("error out"=w961:errorcluster, "value"=w952:string, "found?"=w954:bool, "refnum out"=w958:T5)  [unwired: 3 in]
                n273 = Unbundle By Name(w944) -> ("Permeability"=w953:dbl)
                n274 = Fract/Exp String To Number(string=w952) -> (number=w951:dbl)  [unwired: 3 in, 1 out]
                n275 = Select(t=w951, s=w954, f=w953) -> (s? t:f=w948:dbl)
                n276 = Bundle By Name(cluster=w944, "Permeability"=w948) -> (w955:T2)
                n277 = Not Equal?(x=w948, y=nan) -> (x != y?=w949:bool)
              }
              frame 17 {
                # "Four-pole"
                n278 = call-poly <vilib>:"Read Key.vi"("section"=w963, "error in (no error)"=w978, "default value"=w977, "key"=w974, "refnum"=w975) -> ("error out"=w979:errorcluster, "value"=w969:string, "found?"=w971:bool, "refnum out"=w976:T5)  [unwired: 3 in]
                n279 = Unbundle By Name(w962) -> ("4P"=w970:bool)
                n280 = Equal?(x=w969, y="4P") -> (x = y?=w968:bool)
                n281 = Select(t=w968, s=w971, f=w970) -> (s? t:f=w972:bool)
                n282 = Bundle By Name(cluster=w962, "4P"=w972) -> (w973:T2)
              }
              frame 18 {
                # "Electrode Spacing"
                n283 = call-poly <vilib>:"Read Key.vi"("section"=w981, "error in (no error)"=w996, "default value"=w995, "key"=w992, "refnum"=w993) -> ("error out"=w997:errorcluster, "value"=w988:string, "found?"=w990:bool, "refnum out"=w994:T5)  [unwired: 3 in]
                n284 = Unbundle By Name(w980) -> ("ElectSpace"=w989:dbl)
                n285 = Fract/Exp String To Number(string=w988) -> (number=w987:dbl)  [unwired: 3 in, 1 out]
                n286 = Select(t=w987, s=w990, f=w989) -> (s? t:f=w984:dbl)
                n287 = Bundle By Name(cluster=w980, "ElectSpace"=w984) -> (w991:T2)
                n288 = Not Equal?(x=w984, y=nan) -> (x != y?=w985:bool)
              }
              frame 19 {
                # "Frequency"
                n289 = call-poly <vilib>:"Read Key.vi"("section"=w999, "error in (no error)"=w1014, "default value"=w1013, "key"=w1010, "refnum"=w1011) -> ("error out"=w1015:errorcluster, "value"=w1006:string, "found?"=w1008:bool, "refnum out"=w1012:T5)  [unwired: 3 in]
                n290 = Unbundle By Name(w998) -> ("Frequency"=w1007:dbl)
                n291 = Fract/Exp String To Number(string=w1006) -> (number=w1005:dbl)  [unwired: 3 in, 1 out]
                n292 = Select(t=w1005, s=w1008, f=w1007) -> (s? t:f=w1002:dbl)
                n293 = Bundle By Name(cluster=w998, "Frequency"=w1002) -> (w1009:T2)
                n294 = Not Equal?(x=w1002, y=nan) -> (x != y?=w1003:bool)
              }
              frame 20 {
                # "Amplitude"
                n295 = call-poly <vilib>:"Read Key.vi"("section"=w1017, "error in (no error)"=w1032, "default value"=w1031, "key"=w1028, "refnum"=w1029) -> ("error out"=w1033:errorcluster, "value"=w1024:string, "found?"=w1026:bool, "refnum out"=w1030:T5)  [unwired: 3 in]
                n296 = Unbundle By Name(w1016) -> ("Amplitude"=w1025:dbl)
                n297 = Fract/Exp String To Number(string=w1024) -> (number=w1023:dbl)  [unwired: 3 in, 1 out]
                n298 = Select(t=w1023, s=w1026, f=w1025) -> (s? t:f=w1020:dbl)
                n299 = Bundle By Name(cluster=w1016, "Amplitude"=w1020) -> (w1027:T2)
                n300 = Not Equal?(x=w1020, y=nan) -> (x != y?=w1021:bool)
              }
              frame 21 {
                # "DAQ Period"
                n301 = call-poly <vilib>:"Read Key.vi"("section"=w1035, "error in (no error)"=w1050, "default value"=w1049, "key"=w1046, "refnum"=w1047) -> ("error out"=w1051:errorcluster, "value"=w1041:string, "found?"=w1043:bool, "refnum out"=w1048:T5)  [unwired: 3 in]
                n302 = Unbundle By Name(w1034) -> ("DAQ Period"=w1042:u32)
                n303 = Decimal String To Number(string=w1041, default (0L)=u32 0 ("default (0 I32)")) -> (number=w1040:u32)  [unwired: 1 in, 1 out]
                n304 = Select(t=w1040, s=w1043, f=w1042) -> (s? t:f=w1044:u32)
                n305 = Bundle By Name(cluster=w1034, "DAQ Period"=w1044) -> (w1045:T2)
              }
              frame 22 {
                # "DAQ Units"
                n306 = call-poly <vilib>:"Read Key.vi"("section"=w1053, "error in (no error)"=w1066, "default value"=w1065, "key"=w1062, "refnum"=w1063) -> ("error out"=w1067:errorcluster, "value"=w1060:string, "found?"=w1059:bool, "refnum out"=w1064:T5)  [unwired: 3 in]
                n307 = Unbundle By Name(w1052) -> ("DAQ Units"=w1058:u16)
                n308 = case shown="True" w1059 {
                  tunnel: w1060 -> [_ w1070]
                  tunnel: [w1068 w1069] -> w1057
                  tunnel: w1058 -> [w1068 _]
                  frame False {
                    # "Key not found"
                  }
                  frame True {
                    n309 = case shown="\"Mins\"" w1070 {
                      tunnel: [u16 1 ("DAQ Units") u16 0 ("DAQ Units") u16 1 ("DAQ Units")] -> w1069
                      frame Default {
                      }
                      frame "Mins" {
                      }
                      frame "Hrs" {
                      }
                    }
                  }
                }
                n310 = Bundle By Name(cluster=w1052, "DAQ Units"=w1057) -> (w1061:T2)
              }
              frame 23 {
                # "Start Time"
                n311 = call-poly <vilib>:"Read Key.vi"("section"=w1080, "error in (no error)"=w1094, "default value"=w1093, "key"=w1090, "refnum"=w1091) -> ("error out"=w1095:errorcluster, "value"=w1086:string, "found?"=w1088:bool, "refnum out"=w1092:T5)  [unwired: 3 in]
                n312 = Get Date/Time In Seconds() -> (seconds since 1Jan1904=w1076:timestamp)
                n313 = Unbundle By Name(w1079) -> ("Start Time"=w1087:dbl)
                n314 = Fract/Exp String To Number(string=w1086) -> (number=w1077:dbl)  [unwired: 3 in, 1 out]
                n315 = To Double Precision Float(number=w1076) -> (double precision float=w1075:dbl)
                n316 = Equal To 0?(x=w1077) -> (x = 0?=w1078:bool)
                n317 = Select(t=w1075, s=w1078, f=w1077) -> (s? t:f=w1074:dbl)
                n318 = Select(t=w1074, s=w1088, f=w1087) -> (s? t:f=w1083:dbl)
                n319 = Bundle By Name(cluster=w1079, "Start Time"=w1083) -> (w1089:T2)
                n320 = Not Equal?(x=w1083, y=nan) -> (x != y?=w1084:bool)
              }
              frame 24 {
                # "Next Time"
                n321 = call-poly <vilib>:"Read Key.vi"("section"=w1097, "error in (no error)"=w1112, "default value"=w1111, "key"=w1108, "refnum"=w1109) -> ("error out"=w1113:errorcluster, "value"=w1104:string, "found?"=w1106:bool, "refnum out"=w1110:T5)  [unwired: 3 in]
                n322 = Unbundle By Name(w1096) -> ("Next Time"=w1105:dbl)
                n323 = Fract/Exp String To Number(string=w1104) -> (number=w1103:dbl)  [unwired: 3 in, 1 out]
                n324 = Select(t=w1103, s=w1106, f=w1105) -> (s? t:f=w1100:dbl)
                n325 = Bundle By Name(cluster=w1096, "Next Time"=w1100) -> (w1107:T2)
                n326 = Not Equal?(x=w1100, y=nan) -> (x != y?=w1101:bool)
              }
              frame 25 {
                # "Datafile"
                n327 = call-poly <vilib>:"Read Key.vi"("section"=w1115, "error in (no error)"=w1129, "default value"=w1128, "key"=w1125, "refnum"=w1126) -> ("error out"=w1130:errorcluster, "value"=w1120:string, "found?"=w1122:bool, "refnum out"=w1127:T5)  [unwired: 3 in]
                n328 = Unbundle By Name(w1114) -> ("Datafile"=w1121:path)
                n329 = String To Path(string=w1120) -> (path=w1119:path)
                n330 = Select(t=w1119, s=w1122, f=w1121) -> (s? t:f=w1123:path)
                n331 = Bundle By Name(cluster=w1114, "Datafile"=w1123) -> (w1124:T2)
              }
              frame 26 {
                # "Last Pore Volume"
                n332 = call-poly <vilib>:"Read Key.vi"("section"=w1132, "error in (no error)"=w1147, "default value"=w1146, "key"=w1143, "refnum"=w1144) -> ("error out"=w1148:errorcluster, "value"=w1139:string, "found?"=w1141:bool, "refnum out"=w1145:T5)  [unwired: 3 in]
                n333 = Unbundle By Name(w1131) -> ("Last Pore Vol"=w1140:dbl)
                n334 = Fract/Exp String To Number(string=w1139) -> (number=w1138:dbl)  [unwired: 3 in, 1 out]
                n335 = Select(t=w1138, s=w1141, f=w1140) -> (s? t:f=w1135:dbl)
                n336 = Bundle By Name(cluster=w1131, "Last Pore Vol"=w1135) -> (w1142:T2)
                n337 = Not Equal?(x=w1135, y=nan) -> (x != y?=w1136:bool)
              }
              frame 27 {
                # "Last Pore Xdcr"
                n338 = Unbundle By Name(w1149) -> ("Last Pore Xdcr"=w1157:enum16{"<none>", "Lo Range", "Hi Range"})
                n339 = call-poly <vilib>:"Read Key.vi"("section"=w1150, "error in (no error)"=w1164, "default value"=w1163, "key"=w1160, "refnum"=w1161) -> ("error out"=w1165:errorcluster, "value"=w1152:string, "found?"=w1158:bool, "refnum out"=w1162:T5)  [unwired: 3 in]
                n340 = case shown="\"<none>\", Default" w1152 {
                  tunnel: [enum16{"<none>", "Lo Range", "Hi Range"}."<none>" ("Last Pore Xdcr") enum16{"<none>", "Lo Range", "Hi Range"}."Lo Range" ("Last Pore Xdcr") enum16{"<none>", "Lo Range", "Hi Range"}."Hi Range" ("Last Pore Xdcr")] -> w1151
                  frame "<none>", Default {
                  }
                  frame "Lo Range" {
                  }
                  frame "Hi Range" {
                  }
                }
                n341 = Select(t=w1151, s=w1158, f=w1157) -> (s? t:f=w1156:enum16{"<none>", "Lo Range", "Hi Range"})
                n342 = Bundle By Name(cluster=w1149, "Last Pore Xdcr"=w1156) -> (w1159:T2)
              }
              frame 28 {
                # "Last Resistor"
                n343 = Unbundle By Name(w1169) -> ("Last Resistor"=w1177:T4)
                n344 = call-poly <vilib>:"Read Key.vi"("section"=w1170, "error in (no error)"=w1184, "default value"=w1183, "key"=w1180, "refnum"=w1181) -> ("error out"=w1185:errorcluster, "value"=w1172:string, "found?"=w1178:bool, "refnum out"=w1182:T5)  [unwired: 3 in]
                n345 = case shown="\"Resistor 3\"" w1172 {
                  tunnel: [T4."<none>" ("Last Resistor") T4."Resistor 1" ("Last Resistor") T4."Resistor 2" ("Last Resistor") T4."Resistor 3" ("Last Resistor") T4."Resistor 4" ("Last Resistor") T4."Resistor 5" ("Last Resistor") T4."Resistor 6" ("Last Resistor")] -> w1171
                  frame "<none>", Default {
                  }
                  frame "Resistor 1" {
                  }
                  frame "Resistor 2" {
                  }
                  frame "Resistor 3" {
                  }
                  frame "Resistor 4" {
                  }
                  frame "Resistor 5" {
                  }
                  frame "Resistor 6" {
                  }
                }
                n346 = Select(t=w1171, s=w1178, f=w1177) -> (s? t:f=w1176:T4)
                n347 = Bundle By Name(cluster=w1169, "Last Resistor"=w1176) -> (w1179:T2)
              }
              frame 29 {
                w1199 = 1  # PV Index
                # "ER 1-2"
                n348 = call-poly <vilib>:"Read Key.vi"("section"=w1194, "error in (no error)"=w1209, "default value"=w1208, "key"=w1205, "refnum"=w1206) -> ("error out"=w1210:errorcluster, "value"=w1203:string, "found?"=w1204:bool, "refnum out"=w1207:T5)  [unwired: 3 in]
                n349 = case shown="True" w1204 {
                  tunnel: w1203 -> [_ w1221]
                  tunnel: [TRUE w1219] -> w1202
                  tunnel: [w1211 w1216] -> w1200
                  tunnel: w1196 -> [w1213 _]
                  tunnel: [w1212 w1215] -> w1198
                  tunnel: w1199 -> [w1212 w1215]
                  frame False {
                    n350 = Index Array(array=w1213, index=w1212) -> (element=w1211:dbl)
                  }
                  frame True {
                    n351 = Fract/Exp String To Number(string=w1221) -> (number=w1218:dbl)  [unwired: 3 in, 1 out]
                    n352 = Not Equal?(x=w1218, y=nan) -> (x != y?=w1219:bool)
                    n353 = Select(t=w1218, s=w1219, f=0.0) -> (s? t:f=w1216:dbl)
                  }
                }
                n354 = Replace Array Subset(array=w1195, new element=w1200, index=w1198) -> (w1201:dbl[])
              }
              frame 30 {
                w1227 = 2  # PV Index
                # "ER 1-3"
                n355 = call-poly <vilib>:"Read Key.vi"("section"=w1223, "error in (no error)"=w1238, "default value"=w1237, "key"=w1234, "refnum"=w1235) -> ("error out"=w1239:errorcluster, "value"=w1232:string, "found?"=w1233:bool, "refnum out"=w1236:T5)  [unwired: 3 in]
                n356 = case shown="True" w1233 {
                  tunnel: w1232 -> [_ w1250]
                  tunnel: [TRUE w1248] -> w1231
                  tunnel: [w1240 w1245] -> w1229
                  tunnel: w1224 -> [w1242 _]
                  tunnel: [w1241 w1244] -> w1226
                  tunnel: w1227 -> [w1241 w1244]
                  frame False {
                    n357 = Index Array(array=w1242, index=w1241) -> (element=w1240:dbl)
                  }
                  frame True {
                    n358 = Fract/Exp String To Number(string=w1250) -> (number=w1247:dbl)  [unwired: 3 in, 1 out]
                    n359 = Not Equal?(x=w1247, y=nan) -> (x != y?=w1248:bool)
                    n360 = Select(t=w1247, s=w1248, f=0.0) -> (s? t:f=w1245:dbl)
                  }
                }
                n361 = Replace Array Subset(array=w1228, new element=w1229, index=w1226) -> (w1230:dbl[])
              }
              frame 31 {
                w1257 = 3  # PV Index
                # "ER 1-4"
                n362 = call-poly <vilib>:"Read Key.vi"("section"=w1252, "error in (no error)"=w1267, "default value"=w1266, "key"=w1263, "refnum"=w1264) -> ("error out"=w1268:errorcluster, "value"=w1261:string, "found?"=w1262:bool, "refnum out"=w1265:T5)  [unwired: 3 in]
                n363 = case shown="True" w1262 {
                  tunnel: w1261 -> [_ w1279]
                  tunnel: [TRUE w1277] -> w1260
                  tunnel: [w1269 w1274] -> w1258
                  tunnel: w1254 -> [w1271 _]
                  tunnel: [w1270 w1273] -> w1256
                  tunnel: w1257 -> [w1270 w1273]
                  frame False {
                    n364 = Index Array(array=w1271, index=w1270) -> (element=w1269:dbl)
                  }
                  frame True {
                    n365 = Fract/Exp String To Number(string=w1279) -> (number=w1276:dbl)  [unwired: 3 in, 1 out]
                    n366 = Not Equal?(x=w1276, y=nan) -> (x != y?=w1277:bool)
                    n367 = Select(t=w1276, s=w1277, f=0.0) -> (s? t:f=w1274:dbl)
                  }
                }
                n368 = Replace Array Subset(array=w1253, new element=w1258, index=w1256) -> (w1259:dbl[])
              }
              frame 32 {
                w1286 = 4  # PV Index
                # "ER 2-3"
                n369 = call-poly <vilib>:"Read Key.vi"("section"=w1281, "error in (no error)"=w1296, "default value"=w1295, "key"=w1292, "refnum"=w1293) -> ("error out"=w1297:errorcluster, "value"=w1290:string, "found?"=w1291:bool, "refnum out"=w1294:T5)  [unwired: 3 in]
                n370 = case shown="True" w1291 {
                  tunnel: w1290 -> [_ w1308]
                  tunnel: [TRUE w1306] -> w1289
                  tunnel: [w1298 w1303] -> w1287
                  tunnel: w1283 -> [w1300 _]
                  tunnel: [w1299 w1302] -> w1285
                  tunnel: w1286 -> [w1299 w1302]
                  frame False {
                    n371 = Index Array(array=w1300, index=w1299) -> (element=w1298:dbl)
                  }
                  frame True {
                    n372 = Fract/Exp String To Number(string=w1308) -> (number=w1305:dbl)  [unwired: 3 in, 1 out]
                    n373 = Not Equal?(x=w1305, y=nan) -> (x != y?=w1306:bool)
                    n374 = Select(t=w1305, s=w1306, f=0.0) -> (s? t:f=w1303:dbl)
                  }
                }
                n375 = Replace Array Subset(array=w1282, new element=w1287, index=w1285) -> (w1288:dbl[])
              }
              frame 33 {
                w1315 = 5  # PV Index
                # "FF 2-3"
                n376 = call-poly <vilib>:"Read Key.vi"("section"=w1310, "error in (no error)"=w1325, "default value"=w1324, "key"=w1321, "refnum"=w1322) -> ("error out"=w1326:errorcluster, "value"=w1319:string, "found?"=w1320:bool, "refnum out"=w1323:T5)  [unwired: 3 in]
                n377 = case shown="True" w1320 {
                  tunnel: w1319 -> [_ w1337]
                  tunnel: [TRUE w1335] -> w1318
                  tunnel: [w1327 w1332] -> w1316
                  tunnel: w1312 -> [w1329 _]
                  tunnel: [w1328 w1331] -> w1314
                  tunnel: w1315 -> [w1328 w1331]
                  frame False {
                    n378 = Index Array(array=w1329, index=w1328) -> (element=w1327:dbl)
                  }
                  frame True {
                    n379 = Fract/Exp String To Number(string=w1337) -> (number=w1334:dbl)  [unwired: 3 in, 1 out]
                    n380 = Not Equal?(x=w1334, y=nan) -> (x != y?=w1335:bool)
                    n381 = Select(t=w1334, s=w1335, f=0.0) -> (s? t:f=w1332:dbl)
                  }
                }
                n382 = Replace Array Subset(array=w1311, new element=w1316, index=w1314) -> (w1317:dbl[])
              }
              frame 34 {
                w1343 = 6  # PV Index
                # "Temp A"
                n383 = call-poly <vilib>:"Read Key.vi"("section"=w1339, "error in (no error)"=w1354, "default value"=w1353, "key"=w1350, "refnum"=w1351) -> ("error out"=w1355:errorcluster, "value"=w1348:string, "found?"=w1349:bool, "refnum out"=w1352:T5)  [unwired: 3 in]
                n384 = case shown="True" w1349 {
                  tunnel: w1348 -> [_ w1366]
                  tunnel: [TRUE w1364] -> w1347
                  tunnel: [w1357 w1361] -> w1345
                  tunnel: w1341 -> [w1358 _]
                  tunnel: [w1356 w1360] -> w1342
                  tunnel: w1343 -> [w1356 w1360]
                  frame False {
                    n385 = Index Array(array=w1358, index=w1356) -> (element=w1357:dbl)
                  }
                  frame True {
                    n386 = Fract/Exp String To Number(string=w1366) -> (number=w1363:dbl)  [unwired: 3 in, 1 out]
                    n387 = Not Equal?(x=w1363, y=nan) -> (x != y?=w1364:bool)
                    n388 = Select(t=w1363, s=w1364, f=0.0) -> (s? t:f=w1361:dbl)
                  }
                }
                n389 = Replace Array Subset(array=w1344, new element=w1345, index=w1342) -> (w1346:dbl[])
              }
              frame 35 {
                w1372 = 7  # PV Index
                # "Temp B"
                n390 = call-poly <vilib>:"Read Key.vi"("section"=w1368, "error in (no error)"=w1383, "default value"=w1382, "key"=w1379, "refnum"=w1380) -> ("error out"=w1384:errorcluster, "value"=w1377:string, "found?"=w1378:bool, "refnum out"=w1381:T5)  [unwired: 3 in]
                n391 = case shown="True" w1378 {
                  tunnel: w1377 -> [_ w1395]
                  tunnel: [TRUE w1393] -> w1376
                  tunnel: [w1385 w1390] -> w1374
                  tunnel: w1369 -> [w1387 _]
                  tunnel: [w1386 w1389] -> w1371
                  tunnel: w1372 -> [w1386 w1389]
                  frame False {
                    n392 = Index Array(array=w1387, index=w1386) -> (element=w1385:dbl)
                  }
                  frame True {
                    n393 = Fract/Exp String To Number(string=w1395) -> (number=w1392:dbl)  [unwired: 3 in, 1 out]
                    n394 = Not Equal?(x=w1392, y=nan) -> (x != y?=w1393:bool)
                    n395 = Select(t=w1392, s=w1393, f=0.0) -> (s? t:f=w1390:dbl)
                  }
                }
                n396 = Replace Array Subset(array=w1373, new element=w1374, index=w1371) -> (w1375:dbl[])
              }
              frame 36 {
                w1401 = 8  # PV Index
                # "Conf-P"
                n397 = call-poly <vilib>:"Read Key.vi"("section"=w1397, "error in (no error)"=w1412, "default value"=w1411, "key"=w1408, "refnum"=w1409) -> ("error out"=w1413:errorcluster, "value"=w1406:string, "found?"=w1407:bool, "refnum out"=w1410:T5)  [unwired: 3 in]
                n398 = case shown="True" w1407 {
                  tunnel: w1406 -> [_ w1424]
                  tunnel: [TRUE w1422] -> w1405
                  tunnel: [w1414 w1419] -> w1403
                  tunnel: w1398 -> [w1416 _]
                  tunnel: [w1415 w1418] -> w1400
                  tunnel: w1401 -> [w1415 w1418]
                  frame False {
                    n399 = Index Array(array=w1416, index=w1415) -> (element=w1414:dbl)
                  }
                  frame True {
                    n400 = Fract/Exp String To Number(string=w1424) -> (number=w1421:dbl)  [unwired: 3 in, 1 out]
                    n401 = Not Equal?(x=w1421, y=nan) -> (x != y?=w1422:bool)
                    n402 = Select(t=w1421, s=w1422, f=0.0) -> (s? t:f=w1419:dbl)
                  }
                }
                n403 = Replace Array Subset(array=w1402, new element=w1403, index=w1400) -> (w1404:dbl[])
              }
              frame 37 {
                w1431 = 9  # PV Index
                # "Pore-P"
                n404 = call-poly <vilib>:"Read Key.vi"("section"=w1427, "error in (no error)"=w1441, "default value"=w1440, "key"=w1437, "refnum"=w1438) -> ("error out"=w1442:errorcluster, "value"=w1436:string, "found?"=w1425:bool, "refnum out"=w1439:T5)  [unwired: 3 in]
                n405 = case shown="True" w1425 {
                  tunnel: w1436 -> [_ w1453]
                  tunnel: [TRUE w1451] -> w1435
                  tunnel: [w1443 w1448] -> w1433
                  tunnel: w1428 -> [w1445 _]
                  tunnel: [w1444 w1447] -> w1430
                  tunnel: w1431 -> [w1444 w1447]
                  frame False {
                    n406 = Index Array(array=w1445, index=w1444) -> (element=w1443:dbl)
                  }
                  frame True {
                    n407 = Fract/Exp String To Number(string=w1453) -> (number=w1450:dbl)  [unwired: 3 in, 1 out]
                    n408 = Not Equal?(x=w1450, y=nan) -> (x != y?=w1451:bool)
                    n409 = Select(t=w1450, s=w1451, f=0.0) -> (s? t:f=w1448:dbl)
                  }
                }
                n410 = Replace Array Subset(array=w1432, new element=w1433, index=w1430) -> (w1434:dbl[])
              }
              frame 38 {
                w1460 = 10  # PV Index
                # "Delta-P"
                n411 = call-poly <vilib>:"Read Key.vi"("section"=w1456, "error in (no error)"=w1470, "default value"=w1469, "key"=w1466, "refnum"=w1467) -> ("error out"=w1471:errorcluster, "value"=w1465:string, "found?"=w1454:bool, "refnum out"=w1468:T5)  [unwired: 3 in]
                n412 = case shown="True" w1454 {
                  tunnel: w1465 -> [_ w1482]
                  tunnel: [TRUE w1480] -> w1464
                  tunnel: [w1472 w1477] -> w1462
                  tunnel: w1457 -> [w1474 _]
                  tunnel: [w1473 w1476] -> w1459
                  tunnel: w1460 -> [w1473 w1476]
                  frame False {
                    n413 = Index Array(array=w1474, index=w1473) -> (element=w1472:dbl)
                  }
                  frame True {
                    n414 = Fract/Exp String To Number(string=w1482) -> (number=w1479:dbl)  [unwired: 3 in, 1 out]
                    n415 = Not Equal?(x=w1479, y=nan) -> (x != y?=w1480:bool)
                    n416 = Select(t=w1479, s=w1480, f=0.0) -> (s? t:f=w1477:dbl)
                  }
                }
                n417 = Replace Array Subset(array=w1461, new element=w1462, index=w1459) -> (w1463:dbl[])
              }
              frame 39 {
                w1489 = 11  # PV Index
                # "Downstream Pore Pressure"
                n418 = call-poly <vilib>:"Read Key.vi"("section"=w1485, "error in (no error)"=w1499, "default value"=w1498, "key"=w1495, "refnum"=w1496) -> ("error out"=w1500:errorcluster, "value"=w1494:string, "found?"=w1483:bool, "refnum out"=w1497:T5)  [unwired: 3 in]
                n419 = case shown="True" w1483 {
                  tunnel: w1494 -> [_ w1511]
                  tunnel: [TRUE w1509] -> w1493
                  tunnel: [w1501 w1506] -> w1491
                  tunnel: w1486 -> [w1503 _]
                  tunnel: [w1502 w1505] -> w1488
                  tunnel: w1489 -> [w1502 w1505]
                  frame False {
                    n420 = Index Array(array=w1503, index=w1502) -> (element=w1501:dbl)
                  }
                  frame True {
                    n421 = Fract/Exp String To Number(string=w1511) -> (number=w1508:dbl)  [unwired: 3 in, 1 out]
                    n422 = Not Equal?(x=w1508, y=nan) -> (x != y?=w1509:bool)
                    n423 = Select(t=w1508, s=w1509, f=0.0) -> (s? t:f=w1506:dbl)
                  }
                }
                n424 = Replace Array Subset(array=w1490, new element=w1491, index=w1488) -> (w1492:dbl[])
              }
              frame 40 {
                # "Elapsed time"
                n425 = case shown="False" w1514 {
                  tunnel: w1513 -> [w1525 w1526]
                  tunnel: [w1524 w1526] -> w1512
                  frame False {
                    # "No prev data"
                    n426 = Replace Array Subset(array=w1525, new element=0.0 ("new element/subarray"), index=0) -> (w1524:dbl[])
                  }
                  frame True {
                    # "Already have data"
                  }
                }
              }
              frame 41 {
                # "Last pore vol"
                n427 = case shown="False" w1530 {
                  tunnel: w1529 -> [w1541 w1542]
                  tunnel: [w1540 w1542] -> w1528
                  tunnel: w1527 -> [w1538 _]
                  frame False {
                    # "No prev data"
                    n428 = Unbundle By Name(w1538) -> ("Last Pore Vol"=w1537:dbl)
                    n429 = Replace Array Subset(array=w1541, new element=w1537, index=12) -> (w1540:dbl[])
                  }
                  frame True {
                    # "Already have data"
                  }
                }
              }
              frame 42 {
                # "C14"
                n430 = case shown="False" w1546 {
                  tunnel: w1545 -> [w1556 w1557]
                  tunnel: [w1555 w1557] -> w1544
                  frame False {
                    # "No prev data"
                    n431 = Replace Array Subset(array=w1556, new element=0.0 ("new element/subarray"), index=13) -> (w1555:dbl[])
                  }
                  frame True {
                    # "Already have data"
                  }
                }
              }
              frame 43 {
                # "C23"
                n432 = case shown="False" w1561 {
                  tunnel: w1560 -> [w1571 w1572]
                  tunnel: [w1570 w1572] -> w1559
                  frame False {
                    # "No prev data"
                    n433 = Replace Array Subset(array=w1571, new element=0.0 ("new element/subarray"), index=14) -> (w1570:dbl[])
                  }
                  frame True {
                    # "Already have data"
                  }
                }
              }
            }
            n434 = Compound Arithmetic op=AND(w648, w650, w652) -> (w653:bool)
          }
          n435 = case shown="False" w536 {
            tunnel: [w578 w580] -> w544
            tunnel: w543 -> [_ w580]
            tunnel: w537 -> [w579 _]
            frame False {
              # "No prev data"
              n436 = Build Array(w579) -> (w578:dbl[][])
            }
            frame True {
              # "Use existing data"
            }
          }
          n437 = case shown="True" w564 {
            tunnel: w551 -> [w1577 w1581]
            tunnel: w546 -> [w1575 w1580]
            tunnel: w562 -> [_ w1579]
            frame False {
              # "Key not found"
              n438 = Concatenate Strings("READ CELL STATUS - Key \"" ("Substring"), w1577, "\" in section \"" ("Substring"), w1575, "\" not found !" ("Substring")) -> (w1573:string)
              n439 = One Button Dialog(message=w1573) -> ()  [unwired: 1 in, 1 out]
            }
            frame True {
              n440 = case shown="False" w1579 {
                tunnel: w1581 -> [w1583 _]
                tunnel: w1580 -> [w1582 _]
                frame False {
                  n441 = Concatenate Strings("READ CELL STATUS - Key \"" ("Substring"), w1583, "\" in section \"" ("Substring"), w1582, "\" not a number !" ("Substring")) -> (w1584:string)
                  n442 = One Button Dialog(message=w1584) -> ()  [unwired: 1 in, 1 out]
                }
                frame True {
                  # "Good read"
                }
              }
            }
          }
          n443 = Bundle By Name(cluster=w556, "CurData"=w544, "Comment"="") -> (w557:T2)
          n444 = call <vilib>:"Close Config Data.vi"("error in (no error)"=w571, "write file if changed (T)"=FALSE ("write configuration file? (T)"), "refnum"=w572) -> ("error out"=w573:errorcluster)  [unwired: 7 in, 1 out]
        }
        frame "Write Cell Status" {
          w1588 = T1 {"Title"="", "Version"="", "Last Write"="", "CurCell"=1, "NumCells"=5}  # GenInfoOut
          # "Must be 1-5"
          # "38"
          n445 = Unbundle By Name(w1591) -> ("Cell ID"=w1589:i32)
          n446 = Unbundle By Name(w1591) -> ("CurData"=w1597:dbl[][])
          n447 = Array Size(array=w1593) -> (size(s)=w1602:i32)
          n448 = Index Array(array=w1604, index=w1589) -> (element=w1603:string)
          n449 = Decrement(x=w1602) -> (x-1=w1600:i32)
          n450 = call <vilib>:"Open Config Data (compatibility).vi"("error in (no error)"=w1612, "create file if necessary (T)"=TRUE ("create file if necessary? (T)"), "configuration file path"=w1601) -> ("error out"=w1606:errorcluster, "refnum"=w1605:T5)  [unwired: 6 in, 1 out]
          n451 = Index Array(array=w1597, index (col)=0 ("disabled index (col)")) -> (element=w1598:dbl[])  [unwired: 1 in]
          n452 = Array Size(array=w1598) -> (size(s)=w1596:i32)
          n453 = Decrement(x=w1596) -> (x-1=w1595:i32)
          n454 = Index Array(array=w1597, index (row)=w1595) -> (element=w1594:dbl[])  [unwired: 1 in]
          n455 = while {
            shift-right: [w1624] -> w1608
            shift-left: w1605 -> [w1623]
            shift-right: [w1626] -> w1607
            shift-left: w1606 -> [w1625]
            tunnel: w1603 -> [w1622]
            tunnel: w1593 -> [w1619] mode=indexing
            tunnel: w1600 -> [w1620]
            tunnel: w1594 -> [w1618]
            tunnel: w1592 -> [w1617]
            tunnel: w1591 -> [w1616]
            shift-right: [w1613] -> w1590
            shift-left: w1588 -> [w1614]
            i -> [w1621]
            stop <- w1615 continue-if-true
            n456 = Greater?(x=w1620, y=w1621) -> (0:w1615:bool)
            n457 = case shown="39" w1621 {
              tunnel: [w1634 w1643 w1652 w1665 w1679 w1689 w1702 w1715 w1724 w1733 w1742 w1752 w1762 w1772 w1782 w1792 w1802 w1814 w1824 w1834 w1844 w1854 w1864 w1876 w1886 w1896 w1906 w1916 w1929 w1947 w1958 w1969 w1980 w1991 w2002 w2013 w2024 w2035 w2046 w2057] -> w1626
              tunnel: w1625 -> [w1633 w1642 w1651 w1664 w1678 w1688 w1701 w1714 w1723 w1732 w1741 w1751 w1761 w1771 w1781 w1791 w1801 w1813 w1823 w1833 w1843 w1853 w1863 w1875 w1885 w1895 w1905 w1915 w1928 w1946 w1957 w1968 w1979 w1990 w2001 w2012 w2023 w2034 w2045 w2056]
              tunnel: [w1635 w1644 w1653 w1663 w1677 w1687 w1700 w1713 w1722 w1731 w1740 w1750 w1760 w1770 w1780 w1790 w1800 w1812 w1822 w1832 w1842 w1852 w1862 w1874 w1884 w1894 w1904 w1914 w1927 w1945 w1956 w1967 w1978 w1989 w2000 w2011 w2022 w2033 w2044 w2055] -> w1624
              tunnel: w1623 -> [w1632 w1641 w1650 w1662 w1676 w1686 w1699 w1712 w1721 w1730 w1739 w1749 w1759 w1769 w1779 w1789 w1799 w1811 w1821 w1831 w1841 w1851 w1861 w1873 w1883 w1893 w1903 w1913 w1926 w1944 w1955 w1966 w1977 w1988 w1999 w2010 w2021 w2032 w2043 w2054]
              tunnel: w1622 -> [_ _ _ _ _ w1685 w1698 w1711 w1720 w1729 w1738 w1748 w1758 w1768 w1778 w1788 w1798 w1810 w1820 w1830 w1840 w1850 w1860 w1872 w1882 w1892 w1902 w1912 w1925 w1943 w1954 w1965 w1976 w1987 w1998 w2009 w2020 w2031 w2042 w2053]
              tunnel: w1619 -> [w1630 w1639 w1648 w1661 w1675 w1684 w1697 w1710 w1719 w1728 w1737 w1747 w1757 w1767 w1777 w1787 w1797 w1809 w1819 w1829 w1839 w1849 w1859 w1871 w1881 w1891 w1901 w1911 w1924 w1942 w1953 w1964 w1975 w1986 w1997 w2008 w2019 w2030 w2041 w2052]
              tunnel: w1616 -> [_ _ _ w1660 _ w1683 w1696 w1709 w1718 w1727 w1736 w1746 w1756 w1766 w1776 w1786 w1796 w1808 w1818 w1828 w1838 w1848 w1858 w1870 w1880 w1890 w1900 w1910 w1923 _ _ _ _ _ _ _ _ _ _ _]
              tunnel: w1618 -> [_ _ _ _ _ _ _ _ _ _ _ _ _ _ _ _ _ _ _ _ _ _ _ _ _ _ _ _ _ w1940 w1951 w1962 w1973 w1984 w1995 w2006 w2017 w2028 w2039 w2050]
              tunnel: w1617 -> [_ w1636 _ _ _ _ _ _ _ _ _ _ _ _ _ _ _ _ _ _ _ _ _ _ _ _ _ _ _ _ _ _ _ _ _ _ _ _ _ _]
              tunnel: w1614 -> [w1629 w1638 w1647 w1657 w1674 w1680 w1693 w1707 w1716 w1725 w1734 w1743 w1753 w1763 w1773 w1783 w1793 w1803 w1815 w1825 w1835 w1845 w1855 w1867 w1877 w1887 w1897 w1909 w1922 w1937 w1948 w1959 w1970 w1981 w1992 w2003 w2014 w2025 w2036 w2047]
              tunnel: [w1628 w1637 w1646 w1656 w1673 w1680 w1693 w1707 w1716 w1725 w1734 w1743 w1753 w1763 w1773 w1783 w1793 w1803 w1815 w1825 w1835 w1845 w1855 w1867 w1877 w1887 w1897 w1909 w1922 w1937 w1948 w1959 w1970 w1981 w1992 w2003 w2014 w2025 w2036 w2047] -> w1613
              frame 0, Default {
                w1627 = "Cell Status Data File"
                # "Title"
                n458 = Bundle By Name(cluster=w1629, "Title"=w1627) -> (w1628:T1)
                n459 = call-poly <vilib>:"Write Key.vi"("section"="GenInfo", "error in (no error)"=w1633, "value"=w1627, "key"=w1630, "refnum"=w1632) -> ("error out"=w1634:errorcluster, "refnum out"=w1635:T5)  [unwired: 4 in, 1 out]
              }
              frame 1 {
                # "Version"
                n460 = Bundle By Name(cluster=w1638, "Version"=w1636) -> (w1637:T1)
                n461 = call-poly <vilib>:"Write Key.vi"("section"="GenInfo", "error in (no error)"=w1642, "value"=w1636, "key"=w1639, "refnum"=w1641) -> ("error out"=w1643:errorcluster, "refnum out"=w1644:T5)  [unwired: 4 in, 1 out]
              }
              frame 2 {
                # "Last write time"
                n462 = Get Date/Time String() -> (date string=w1645:string)  [unwired: 3 in, 1 out]
                n463 = Bundle By Name(cluster=w1647, "Last Write"=w1645) -> (w1646:T1)
                n464 = call-poly <vilib>:"Write Key.vi"("section"="GenInfo", "error in (no error)"=w1651, "value"=w1645, "key"=w1648, "refnum"=w1650) -> ("error out"=w1652:errorcluster, "refnum out"=w1653:T5)  [unwired: 4 in, 1 out]
              }
              frame 3 {
                # "Currrent Cell"
                n465 = Unbundle By Name(w1660) -> ("Cell ID"=w1659:i32)
                n466 = case shown="0, Default" w1659 {
                  selector: w1659 -> [_ w1669]
                  tunnel: ["1" w1668] -> w1658
                  tunnel: [1 w1669] -> w1655
                  frame 0, Default {
                  }
                  frame 1..5 {
                    n467 = Number To Decimal String(number=w1669) -> (decimal integer string=w1668:string)  [unwired: 1 in]
                  }
                }
                n468 = Bundle By Name(cluster=w1657, "CurCell"=w1655) -> (w1656:T1)
                n469 = call-poly <vilib>:"Write Key.vi"("section"="GenInfo", "error in (no error)"=w1664, "value"=w1658, "key"=w1661, "refnum"=w1662) -> ("error out"=w1665:errorcluster, "refnum out"=w1663:T5)  [unwired: 4 in, 1 out]
              }
              frame 4 {
                # "Number of cells"
                n470 = Bundle By Name(cluster=w1674, "NumCells"=5) -> (w1673:T1)
                n471 = call-poly <vilib>:"Write Key.vi"("section"="GenInfo", "error in (no error)"=w1678, "value"="5", "key"=w1675, "refnum"=w1676) -> ("error out"=w1679:errorcluster, "refnum out"=w1677:T5)  [unwired: 4 in, 1 out]
              }
              frame 5 {
                # "Cell ID"
                n472 = Unbundle By Name(w1683) -> ("Cell ID"=w1682:i32)
                n473 = case shown="0, Default" w1682 {
                  selector: w1682 -> [_ w1692]
                  tunnel: ["1" w1691] -> w1681
                  frame 0, Default {
                  }
                  frame 1..5 {
                    n474 = Number To Decimal String(number=w1692) -> (decimal integer string=w1691:string)  [unwired: 1 in]
                  }
                }
                n475 = call-poly <vilib>:"Write Key.vi"("section"=w1685, "error in (no error)"=w1688, "value"=w1681, "key"=w1684, "refnum"=w1686) -> ("error out"=w1689:errorcluster, "refnum out"=w1687:T5)  [unwired: 4 in, 1 out]
              }
              frame 6 {
                # "Cell Status"
                n476 = Unbundle By Name(w1696) -> ("Cell Status"=w1695:enum16{"Inactive", "Setup", "Active", "Done"})
                n477 = case shown="\"Inactive\", Default" w1695 {
                  tunnel: ["Inactive" "Setup" "Active" "Done"] -> w1694
                  frame "Inactive", Default {
                  }
                  frame "Setup" {
                  }
                  frame "Active" {
                  }
                  frame "Done" {
                  }
                }
                n478 = call-poly <vilib>:"Write Key.vi"("section"=w1698, "error in (no error)"=w1701, "value"=w1694, "key"=w1697, "refnum"=w1699) -> ("error out"=w1702:errorcluster, "refnum out"=w1700:T5)  [unwired: 4 in, 1 out]
              }
              frame 7 {
                # "Project"
                n479 = Unbundle By Name(w1709) -> ("Project"=w1708:string)
                n480 = call-poly <vilib>:"Write Key.vi"("section"=w1711, "error in (no error)"=w1714, "value"=w1708, "key"=w1710, "refnum"=w1712) -> ("error out"=w1715:errorcluster, "refnum out"=w1713:T5)  [unwired: 4 in, 1 out]
              }
              frame 8 {
                # "Sample ID"
                n481 = Unbundle By Name(w1718) -> ("Sample #"=w1717:string)
                n482 = call-poly <vilib>:"Write Key.vi"("section"=w1720, "error in (no error)"=w1723, "value"=w1717, "key"=w1719, "refnum"=w1721) -> ("error out"=w1724:errorcluster, "refnum out"=w1722:T5)  [unwired: 4 in, 1 out]
              }
              frame 9 {
                # "Rock Type"
                n483 = Unbundle By Name(w1727) -> ("Rock Type"=w1726:string)
                n484 = call-poly <vilib>:"Write Key.vi"("section"=w1729, "error in (no error)"=w1732, "value"=w1726, "key"=w1728, "refnum"=w1730) -> ("error out"=w1733:errorcluster, "refnum out"=w1731:T5)  [unwired: 4 in, 1 out]
              }
              frame 10 {
                # "Fluid Pair"
                n485 = Unbundle By Name(w1736) -> ("Fluid Pair"=w1735:string)
                n486 = call-poly <vilib>:"Write Key.vi"("section"=w1738, "error in (no error)"=w1741, "value"=w1735, "key"=w1737, "refnum"=w1739) -> ("error out"=w1742:errorcluster, "refnum out"=w1740:T5)  [unwired: 4 in, 1 out]
              }
              frame 11 {
                # "Rw"
                n487 = Unbundle By Name(w1746) -> ("Rw"=w1745:dbl)
                n488 = Number To Fractional String(number=w1745) -> (F-format string=w1744:string)  [unwired: 3 in]
                n489 = call-poly <vilib>:"Write Key.vi"("section"=w1748, "error in (no error)"=w1751, "value"=w1744, "key"=w1747, "refnum"=w1749) -> ("error out"=w1752:errorcluster, "refnum out"=w1750:T5)  [unwired: 4 in, 1 out]
              }
              frame 12 {
                # "Rw Temperature"
                n490 = Unbundle By Name(w1756) -> ("Rw Temp"=w1755:dbl)
                n491 = Number To Fractional String(number=w1755) -> (F-format string=w1754:string)  [unwired: 3 in]
                n492 = call-poly <vilib>:"Write Key.vi"("section"=w1758, "error in (no error)"=w1761, "value"=w1754, "key"=w1757, "refnum"=w1759) -> ("error out"=w1762:errorcluster, "refnum out"=w1760:T5)  [unwired: 4 in, 1 out]
              }
              frame 13 {
                # "Sample Length"
                n493 = Unbundle By Name(w1766) -> ("Length"=w1765:dbl)
                n494 = Number To Fractional String(number=w1765) -> (F-format string=w1764:string)  [unwired: 3 in]
                n495 = call-poly <vilib>:"Write Key.vi"("section"=w1768, "error in (no error)"=w1771, "value"=w1764, "key"=w1767, "refnum"=w1769) -> ("error out"=w1772:errorcluster, "refnum out"=w1770:T5)  [unwired: 4 in, 1 out]
              }
              frame 14 {
                # "Sample Diameter"
                n496 = Unbundle By Name(w1776) -> ("Diameter"=w1775:dbl)
                n497 = Number To Fractional String(number=w1775) -> (F-format string=w1774:string)  [unwired: 3 in]
                n498 = call-poly <vilib>:"Write Key.vi"("section"=w1778, "error in (no error)"=w1781, "value"=w1774, "key"=w1777, "refnum"=w1779) -> ("error out"=w1782:errorcluster, "refnum out"=w1780:T5)  [unwired: 4 in, 1 out]
              }
              frame 15 {
                # "Porosity"
                n499 = Unbundle By Name(w1786) -> ("Porosity"=w1785:dbl)
                n500 = Number To Fractional String(number=w1785) -> (F-format string=w1784:string)  [unwired: 3 in]
                n501 = call-poly <vilib>:"Write Key.vi"("section"=w1788, "error in (no error)"=w1791, "value"=w1784, "key"=w1787, "refnum"=w1789) -> ("error out"=w1792:errorcluster, "refnum out"=w1790:T5)  [unwired: 4 in, 1 out]
              }
              frame 16 {
                # "Permeability"
                n502 = Unbundle By Name(w1796) -> ("Permeability"=w1795:dbl)
                n503 = Number To Fractional String(number=w1795) -> (F-format string=w1794:string)  [unwired: 3 in]
                n504 = call-poly <vilib>:"Write Key.vi"("section"=w1798, "error in (no error)"=w1801, "value"=w1794, "key"=w1797, "refnum"=w1799) -> ("error out"=w1802:errorcluster, "refnum out"=w1800:T5)  [unwired: 4 in, 1 out]
              }
              frame 17 {
                # "2P/4P"
                n505 = Unbundle By Name(w1808) -> ("4P"=w1807:bool)
                n506 = Select(t="4P" ("y"), s=w1807, f="2P" ("y")) -> (s? t:f=w1804:string)
                n507 = call-poly <vilib>:"Write Key.vi"("section"=w1810, "error in (no error)"=w1813, "value"=w1804, "key"=w1809, "refnum"=w1811) -> ("error out"=w1814:errorcluster, "refnum out"=w1812:T5)  [unwired: 4 in, 1 out]
              }
              frame 18 {
                # "Electrode Spacing"
                n508 = Unbundle By Name(w1818) -> ("ElectSpace"=w1817:dbl)
                n509 = Number To Fractional String(number=w1817) -> (F-format string=w1816:string)  [unwired: 3 in]
                n510 = call-poly <vilib>:"Write Key.vi"("section"=w1820, "error in (no error)"=w1823, "value"=w1816, "key"=w1819, "refnum"=w1821) -> ("error out"=w1824:errorcluster, "refnum out"=w1822:T5)  [unwired: 4 in, 1 out]
              }
              frame 19 {
                # "Frequency"
                n511 = Unbundle By Name(w1828) -> ("Frequency"=w1827:dbl)
                n512 = Number To Fractional String(number=w1827) -> (F-format string=w1826:string)  [unwired: 3 in]
                n513 = call-poly <vilib>:"Write Key.vi"("section"=w1830, "error in (no error)"=w1833, "value"=w1826, "key"=w1829, "refnum"=w1831) -> ("error out"=w1834:errorcluster, "refnum out"=w1832:T5)  [unwired: 4 in, 1 out]
              }
              frame 20 {
                # "Amplitude"
                n514 = Unbundle By Name(w1838) -> ("Amplitude"=w1837:dbl)
                n515 = Number To Fractional String(number=w1837) -> (F-format string=w1836:string)  [unwired: 3 in]
                n516 = call-poly <vilib>:"Write Key.vi"("section"=w1840, "error in (no error)"=w1843, "value"=w1836, "key"=w1839, "refnum"=w1841) -> ("error out"=w1844:errorcluster, "refnum out"=w1842:T5)  [unwired: 4 in, 1 out]
              }
              frame 21 {
                # "DAQ Period"
                n517 = Unbundle By Name(w1848) -> ("DAQ Period"=w1847:u32)
                n518 = Number To Decimal String(number=w1847) -> (decimal integer string=w1846:string)  [unwired: 1 in]
                n519 = call-poly <vilib>:"Write Key.vi"("section"=w1850, "error in (no error)"=w1853, "value"=w1846, "key"=w1849, "refnum"=w1851) -> ("error out"=w1854:errorcluster, "refnum out"=w1852:T5)  [unwired: 4 in, 1 out]
              }
              frame 22 {
                # "DAQ Units"
                n520 = Unbundle By Name(w1858) -> ("DAQ Units"=w1857:u16)
                n521 = case shown="1" w1857 {
                  tunnel: ["Mins" "Hrs"] -> w1856
                  frame 0, Default {
                  }
                  frame 1 {
                  }
                }
                n522 = call-poly <vilib>:"Write Key.vi"("section"=w1860, "error in (no error)"=w1863, "value"=w1856, "key"=w1859, "refnum"=w1861) -> ("error out"=w1864:errorcluster, "refnum out"=w1862:T5)  [unwired: 4 in, 1 out]
              }
              frame 23 {
                # "Start TIme"
                n523 = Unbundle By Name(w1870) -> ("Start Time"=w1869:dbl)
                n524 = Number To Fractional String(number=w1869) -> (F-format string=w1868:string)  [unwired: 3 in]
                n525 = call-poly <vilib>:"Write Key.vi"("section"=w1872, "error in (no error)"=w1875, "value"=w1868, "key"=w1871, "refnum"=w1873) -> ("error out"=w1876:errorcluster, "refnum out"=w1874:T5)  [unwired: 4 in, 1 out]
              }
              frame 24 {
                # "Next Time"
                n526 = Unbundle By Name(w1880) -> ("Next Time"=w1879:dbl)
                n527 = Number To Fractional String(number=w1879) -> (F-format string=w1878:string)  [unwired: 3 in]
                n528 = call-poly <vilib>:"Write Key.vi"("section"=w1882, "error in (no error)"=w1885, "value"=w1878, "key"=w1881, "refnum"=w1883) -> ("error out"=w1886:errorcluster, "refnum out"=w1884:T5)  [unwired: 4 in, 1 out]
              }
              frame 25 {
                # "Data File"
                n529 = Unbundle By Name(w1890) -> ("Datafile"=w1889:path)
                n530 = Path To String(path=w1889) -> (string=w1888:string)
                n531 = call-poly <vilib>:"Write Key.vi"("section"=w1892, "error in (no error)"=w1895, "value"=w1888, "key"=w1891, "refnum"=w1893) -> ("error out"=w1896:errorcluster, "refnum out"=w1894:T5)  [unwired: 4 in, 1 out]
              }
              frame 26 {
                # "Pore Volume"
                n532 = Unbundle By Name(w1900) -> ("Last Pore Vol"=w1899:dbl)
                n533 = Number To Fractional String(number=w1899) -> (F-format string=w1898:string)  [unwired: 3 in]
                n534 = call-poly <vilib>:"Write Key.vi"("section"=w1902, "error in (no error)"=w1905, "value"=w1898, "key"=w1901, "refnum"=w1903) -> ("error out"=w1906:errorcluster, "refnum out"=w1904:T5)  [unwired: 4 in, 1 out]
              }
              frame 27 {
                # "Last Resistor"
                n535 = Unbundle By Name(w1910) -> ("Last Pore Xdcr"=w1908:enum16{"<none>", "Lo Range", "Hi Range"})
                n536 = case shown="\"<none>\", Default" w1908 {
                  tunnel: ["<none>" "Lo Range" "Hi Range"] -> w1907
                  frame "<none>", Default {
                  }
                  frame "Lo Range" {
                  }
                  frame "Hi Range" {
                  }
                }
                n537 = call-poly <vilib>:"Write Key.vi"("section"=w1912, "error in (no error)"=w1915, "value"=w1907, "key"=w1911, "refnum"=w1913) -> ("error out"=w1916:errorcluster, "refnum out"=w1914:T5)  [unwired: 4 in, 1 out]
              }
              frame 28 {
                # "Last Resistor"
                n538 = Unbundle By Name(w1923) -> ("Last Resistor"=w1921:T4)
                n539 = case shown="\"Resistor 6\"" w1921 {
                  tunnel: ["<none>" "Resistor 1" "Resistor 2" "Resistor 3" "Resistor 4" "Resistor 5" "Resistor 6"] -> w1920
                  frame "<none>", Default {
                  }
                  frame "Resistor 1" {
                  }
                  frame "Resistor 2" {
                  }
                  frame "Resistor 3" {
                  }
                  frame "Resistor 4" {
                  }
                  frame "Resistor 5" {
                  }
                  frame "Resistor 6" {
                  }
                }
                n540 = call-poly <vilib>:"Write Key.vi"("section"=w1925, "error in (no error)"=w1928, "value"=w1920, "key"=w1924, "refnum"=w1926) -> ("error out"=w1929:errorcluster, "refnum out"=w1927:T5)  [unwired: 4 in, 1 out]
              }
              frame 29 {
                w1941 = 1  # PV Index
                # "ER 1-2"
                n541 = Index Array(array=w1940, index=w1941) -> (element=w1939:dbl)
                n542 = Number To Fractional String(number=w1939) -> (F-format string=w1938:string)  [unwired: 3 in]
                n543 = call-poly <vilib>:"Write Key.vi"("section"=w1943, "error in (no error)"=w1946, "value"=w1938, "key"=w1942, "refnum"=w1944) -> ("error out"=w1947:errorcluster, "refnum out"=w1945:T5)  [unwired: 4 in, 1 out]
              }
              frame 30 {
                w1952 = 2  # PV Index
                # "ER 1-3"
                n544 = Index Array(array=w1951, index=w1952) -> (element=w1950:dbl)
                n545 = Number To Fractional String(number=w1950) -> (F-format string=w1949:string)  [unwired: 3 in]
                n546 = call-poly <vilib>:"Write Key.vi"("section"=w1954, "error in (no error)"=w1957, "value"=w1949, "key"=w1953, "refnum"=w1955) -> ("error out"=w1958:errorcluster, "refnum out"=w1956:T5)  [unwired: 4 in, 1 out]
              }
              frame 31 {
                w1963 = 3  # PV Index
                # "ER 1-4"
                n547 = Index Array(array=w1962, index=w1963) -> (element=w1961:dbl)
                n548 = Number To Fractional String(number=w1961) -> (F-format string=w1960:string)  [unwired: 3 in]
                n549 = call-poly <vilib>:"Write Key.vi"("section"=w1965, "error in (no error)"=w1968, "value"=w1960, "key"=w1964, "refnum"=w1966) -> ("error out"=w1969:errorcluster, "refnum out"=w1967:T5)  [unwired: 4 in, 1 out]
              }
              frame 32 {
                w1974 = 4  # PV Index
                # "ER 2-3"
                n550 = Index Array(array=w1973, index=w1974) -> (element=w1972:dbl)
                n551 = Number To Fractional String(number=w1972) -> (F-format string=w1971:string)  [unwired: 3 in]
                n552 = call-poly <vilib>:"Write Key.vi"("section"=w1976, "error in (no error)"=w1979, "value"=w1971, "key"=w1975, "refnum"=w1977) -> ("error out"=w1980:errorcluster, "refnum out"=w1978:T5)  [unwired: 4 in, 1 out]
              }
              frame 33 {
                w1985 = 5  # PV Index
                # "FF 2-3"
                n553 = Index Array(array=w1984, index=w1985) -> (element=w1983:dbl)
                n554 = Number To Fractional String(number=w1983) -> (F-format string=w1982:string)  [unwired: 3 in]
                n555 = call-poly <vilib>:"Write Key.vi"("section"=w1987, "error in (no error)"=w1990, "value"=w1982, "key"=w1986, "refnum"=w1988) -> ("error out"=w1991:errorcluster, "refnum out"=w1989:T5)  [unwired: 4 in, 1 out]
              }
              frame 34 {
                w1996 = 6  # PV Index
                # "Temp A"
                n556 = Index Array(array=w1995, index=w1996) -> (element=w1994:dbl)
                n557 = Number To Fractional String(number=w1994) -> (F-format string=w1993:string)  [unwired: 3 in]
                n558 = call-poly <vilib>:"Write Key.vi"("section"=w1998, "error in (no error)"=w2001, "value"=w1993, "key"=w1997, "refnum"=w1999) -> ("error out"=w2002:errorcluster, "refnum out"=w2000:T5)  [unwired: 4 in, 1 out]
              }
              frame 35 {
                w2007 = 7  # PV Index
                # "Temp B"
                n559 = Index Array(array=w2006, index=w2007) -> (element=w2005:dbl)
                n560 = Number To Fractional String(number=w2005) -> (F-format string=w2004:string)  [unwired: 3 in]
                n561 = call-poly <vilib>:"Write Key.vi"("section"=w2009, "error in (no error)"=w2012, "value"=w2004, "key"=w2008, "refnum"=w2010) -> ("error out"=w2013:errorcluster, "refnum out"=w2011:T5)  [unwired: 4 in, 1 out]
              }
              frame 36 {
                w2018 = 8  # PV Index
                # "Conf-P"
                n562 = Index Array(array=w2017, index=w2018) -> (element=w2016:dbl)
                n563 = Number To Fractional String(number=w2016) -> (F-format string=w2015:string)  [unwired: 3 in]
                n564 = call-poly <vilib>:"Write Key.vi"("section"=w2020, "error in (no error)"=w2023, "value"=w2015, "key"=w2019, "refnum"=w2021) -> ("error out"=w2024:errorcluster, "refnum out"=w2022:T5)  [unwired: 4 in, 1 out]
              }
              frame 37 {
                w2029 = 9  # PV Index
                # "Pore-P"
                n565 = Index Array(array=w2028, index=w2029) -> (element=w2027:dbl)
                n566 = Number To Fractional String(number=w2027) -> (F-format string=w2026:string)  [unwired: 3 in]
                n567 = call-poly <vilib>:"Write Key.vi"("section"=w2031, "error in (no error)"=w2034, "value"=w2026, "key"=w2030, "refnum"=w2032) -> ("error out"=w2035:errorcluster, "refnum out"=w2033:T5)  [unwired: 4 in, 1 out]
              }
              frame 38 {
                w2040 = 10  # PV Index
                # "Delta Press"
                n568 = Index Array(array=w2039, index=w2040) -> (element=w2038:dbl)
                n569 = Number To Fractional String(number=w2038) -> (F-format string=w2037:string)  [unwired: 3 in]
                n570 = call-poly <vilib>:"Write Key.vi"("section"=w2042, "error in (no error)"=w2045, "value"=w2037, "key"=w2041, "refnum"=w2043) -> ("error out"=w2046:errorcluster, "refnum out"=w2044:T5)  [unwired: 4 in, 1 out]
              }
              frame 39 {
                w2051 = 11  # PV Index
                # "Downstream Pore Pressure"
                n571 = Index Array(array=w2050, index=w2051) -> (element=w2049:dbl)
                n572 = Number To Fractional String(number=w2049) -> (F-format string=w2048:string)  [unwired: 3 in]
                n573 = call-poly <vilib>:"Write Key.vi"("section"=w2053, "error in (no error)"=w2056, "value"=w2048, "key"=w2052, "refnum"=w2054) -> ("error out"=w2057:errorcluster, "refnum out"=w2055:T5)  [unwired: 4 in, 1 out]
              }
            }
          }
          n574 = call <vilib>:"Close Config Data.vi"("error in (no error)"=w1607, "write file if changed (T)"=TRUE ("write configuration file? (T)"), "refnum"=w1608) -> ("error out"=w1609:errorcluster)  [unwired: 7 in, 1 out]
        }
      }
    }
    frame True {
      w2058 = T1 {"Title"="", "Version"="", "Last Write"="", "CurCell"=1, "NumCells"=5}  # GenInfoOut
      # "Previous error"
    }
  }
  "ErrorOut" <- w14
  "FilePathOut" <- w7
  "Cell x Data Out" <- w4
  "GenInfoOut" <- w1
